vi "ScanningWaveform_v4.vi"(0 "Vy-min":dbl, 1 "Vy-max":dbl, 2 "yPixels/tPixels":dbl, 3 "xPixels/rPixels":dbl, 4 "Vx-min":dbl, 5 "Vx-max":dbl, 6 "Drawing Mode":u16(ring) items=["Image", "Fill Rectangle", "Fill Circle", "Draw Freeform", "Fill Freeform", "Ellipse Boundary", "Line"], 7 "Angle":dbl, 8 "Scanning Mode":u16(ring) items=["Raster", "Spiral"], 9 "AOrate":dbl, 10 "Points":cluster{"X":dbl, "Y":dbl}[](array[cluster]), 11 "points in ellipse":dbl) -> (12 "numPixels":dbl, 13 "Y-WaveArray":dbl[](array[numeric]), 14 "P":dbl, 19 "X-WaveArray":dbl[](array[numeric]))   [LabVIEW 2015]
uses:
  <vilib>/measure/NI_MABase.lvlib
panel:
  out "error IO":errorcluster
  out "Y Graph 4":dbl[][](graph)
  out "Y Graph 3":dbl[][](graph)
  out "X-Y Graph 3":T1(graph)
  out "Y Graph 2":dbl[](graph)
  out "X-Y Graph 2":cluster{dbl[], dbl[]}(graph)
  out "min":dbl
  out "max":dbl
  out "Points 2":cluster{"R":dbl, "Theta":dbl}[](array[cluster])
  out "X-Y Graph":cluster{dbl[], dbl[]}(graph)
  out "flyback time (us)":dbl
  out "Y Graph":dbl[](graph)
  out "X Graph":dbl[](graph)
  out "C":dbl
  out "Sx":dbl
  out "S":dbl
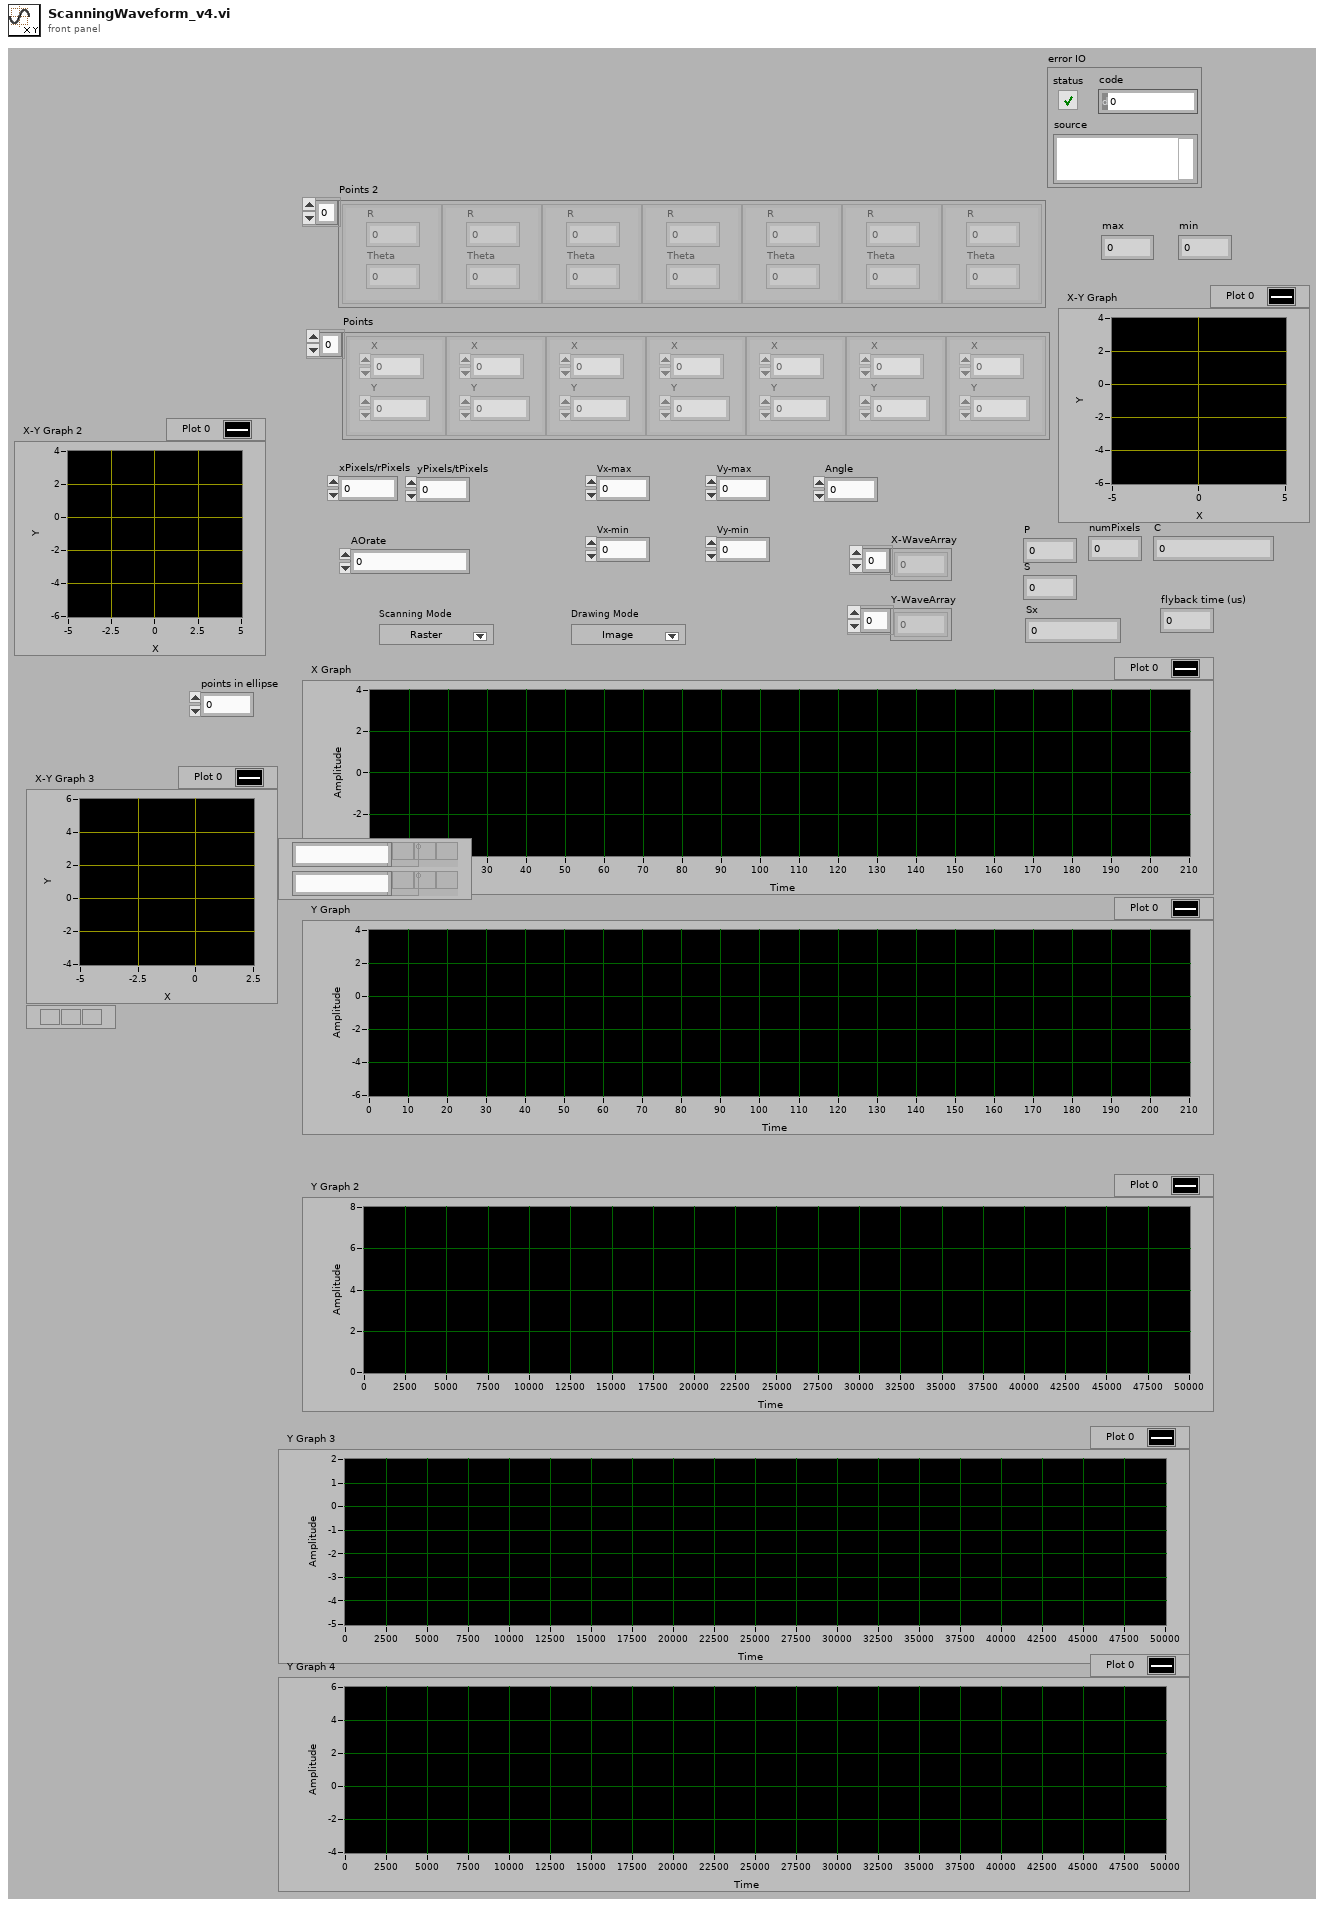
[diagram p1: front panel]
types:
  T1 = cluster{"X-WaveArray":dbl[], "Y-WaveArray":dbl[]}[]
  T2 = typedef "LVRectTypeDef.ctl" = cluster{"Left":i16, "Top":i16, "Right":i16, "Bottom":i16}
  T3 = cluster{"Xpixels":i32, "Vxminref":dbl, "Vxmaxref":dbl, "P":dbl, "Ypixels":i32, "Vyminref":dbl, "Vymaxref":dbl, "srate":sgl, "sAOxy":i32, "timeout":dbl, "type":string, "date":string, "time":string, "Colormap":u16, "Drawing Mode":u16, "Scanning Mode":u16, "square pixels":bool, "square matrix":bool, "Xpixels Img":i32, "Vx-min Img":dbl, "VX-max Img":dbl, "Ypixels Img":i32, "Vy-min Img":dbl, "Vy-max Img ":dbl, "Angle Img":dbl, "autoshutter":bool, "finite":bool, "cont":bool, "wavdet":bool, "measpoints":i32, "avpp":i32, "bufferAO":i32, "bufferAI":i32, "starttick":u32, "waveform":path, "Vx-ref":dbl, "Vy-ref":dbl, "refreshrate":dbl, "refreshbuffer":i32, "tt_cycles":i32, "motorref":refnum<k7>, "mirrorswitch":refnum<k7>, "sample mode":i32, "maxbufferAI":i32, "srateAODO":sgl, "bin":sgl, "Pel":sgl, "Angle draw":dbl, "srate Img":sgl, "ROIimg_plotbounds":T2, "auto OD":bool, "ODfilt":u16, "aAI":i32[], "aCI":i32[], "aAO":u32[], "aDO":u32[], "refwfsize":dbl, "Lifetime":bool, "Vz-Img":dbl, "Vz-ref":dbl, "Vz-reset":dbl, "AIoverride":bool, "aAS":u32[], "XYZstart":dbl[]}
  T4 = cluster{cluster{dbl, dbl}[], cluster{dbl, dbl}[]}
  T5 = cluster{"X-WaveArray":dbl[], "Y-WaveArray":dbl[]}
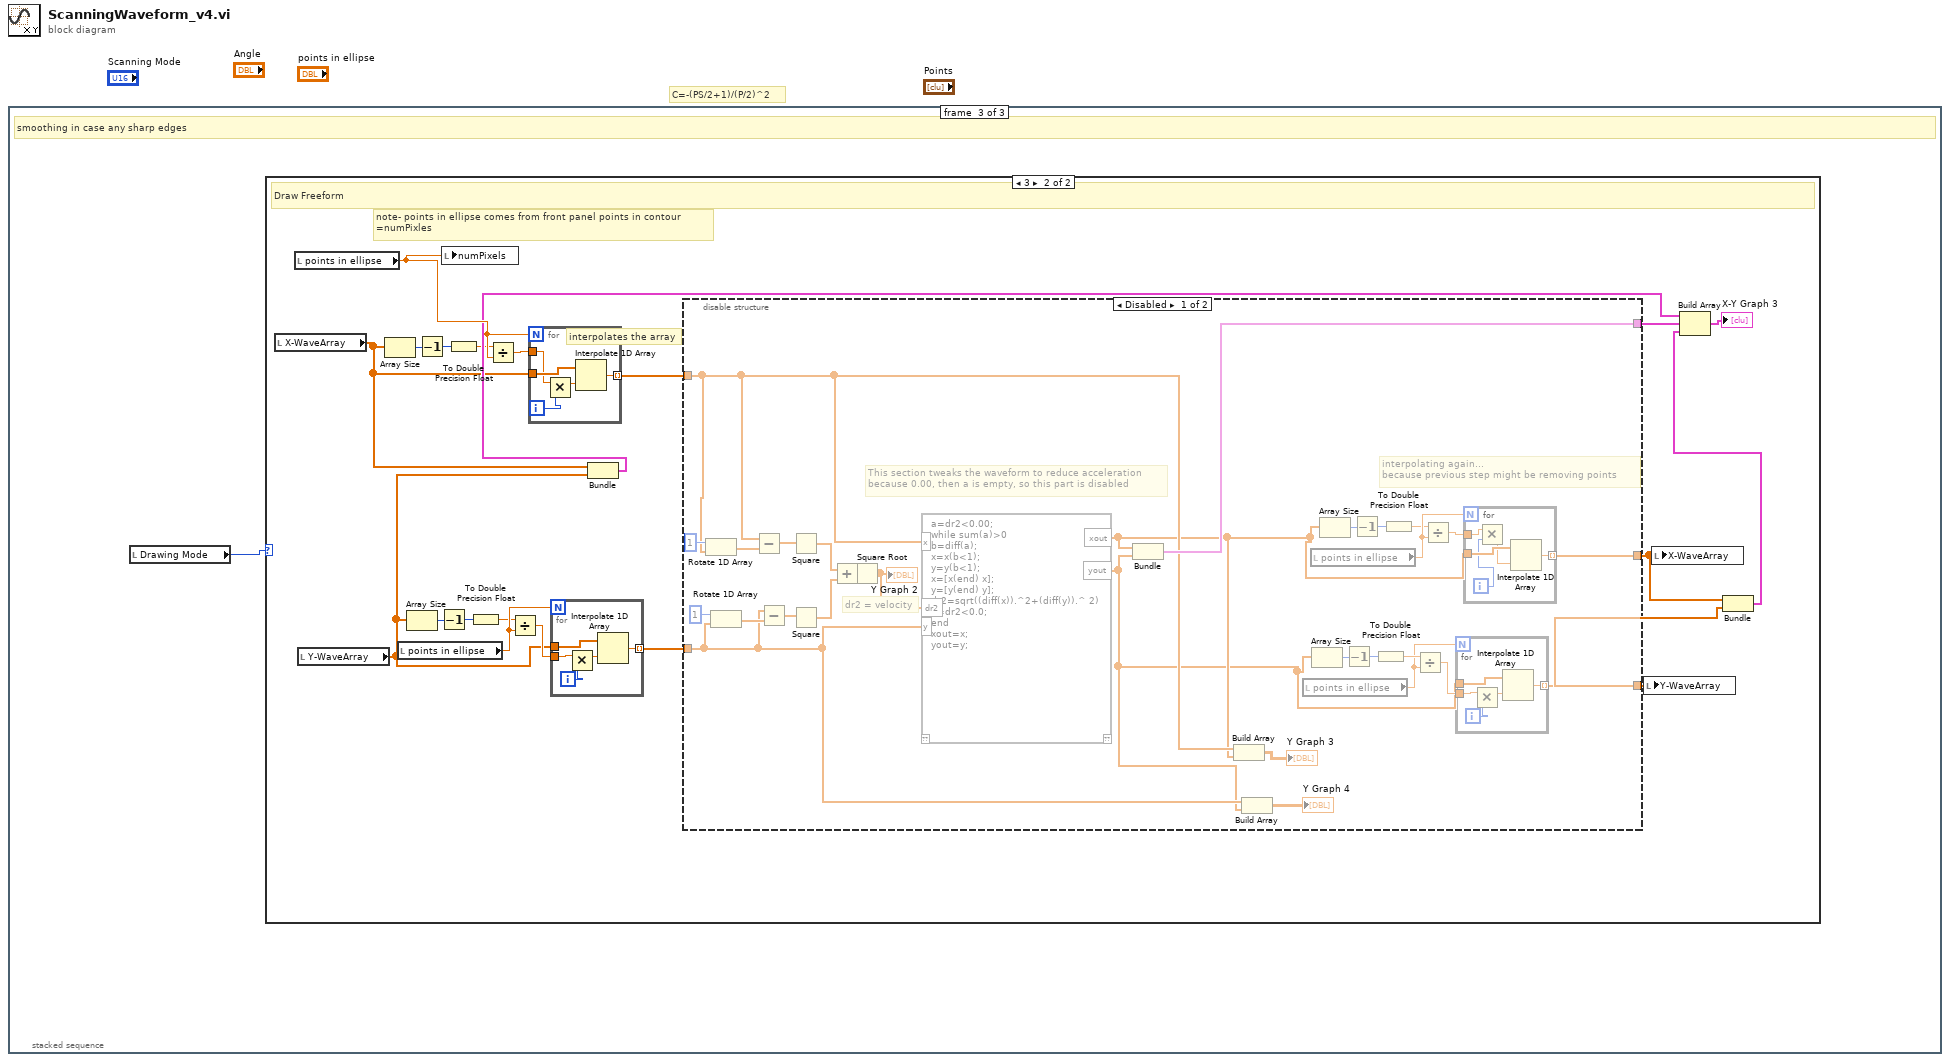
[diagram p0: block diagram]
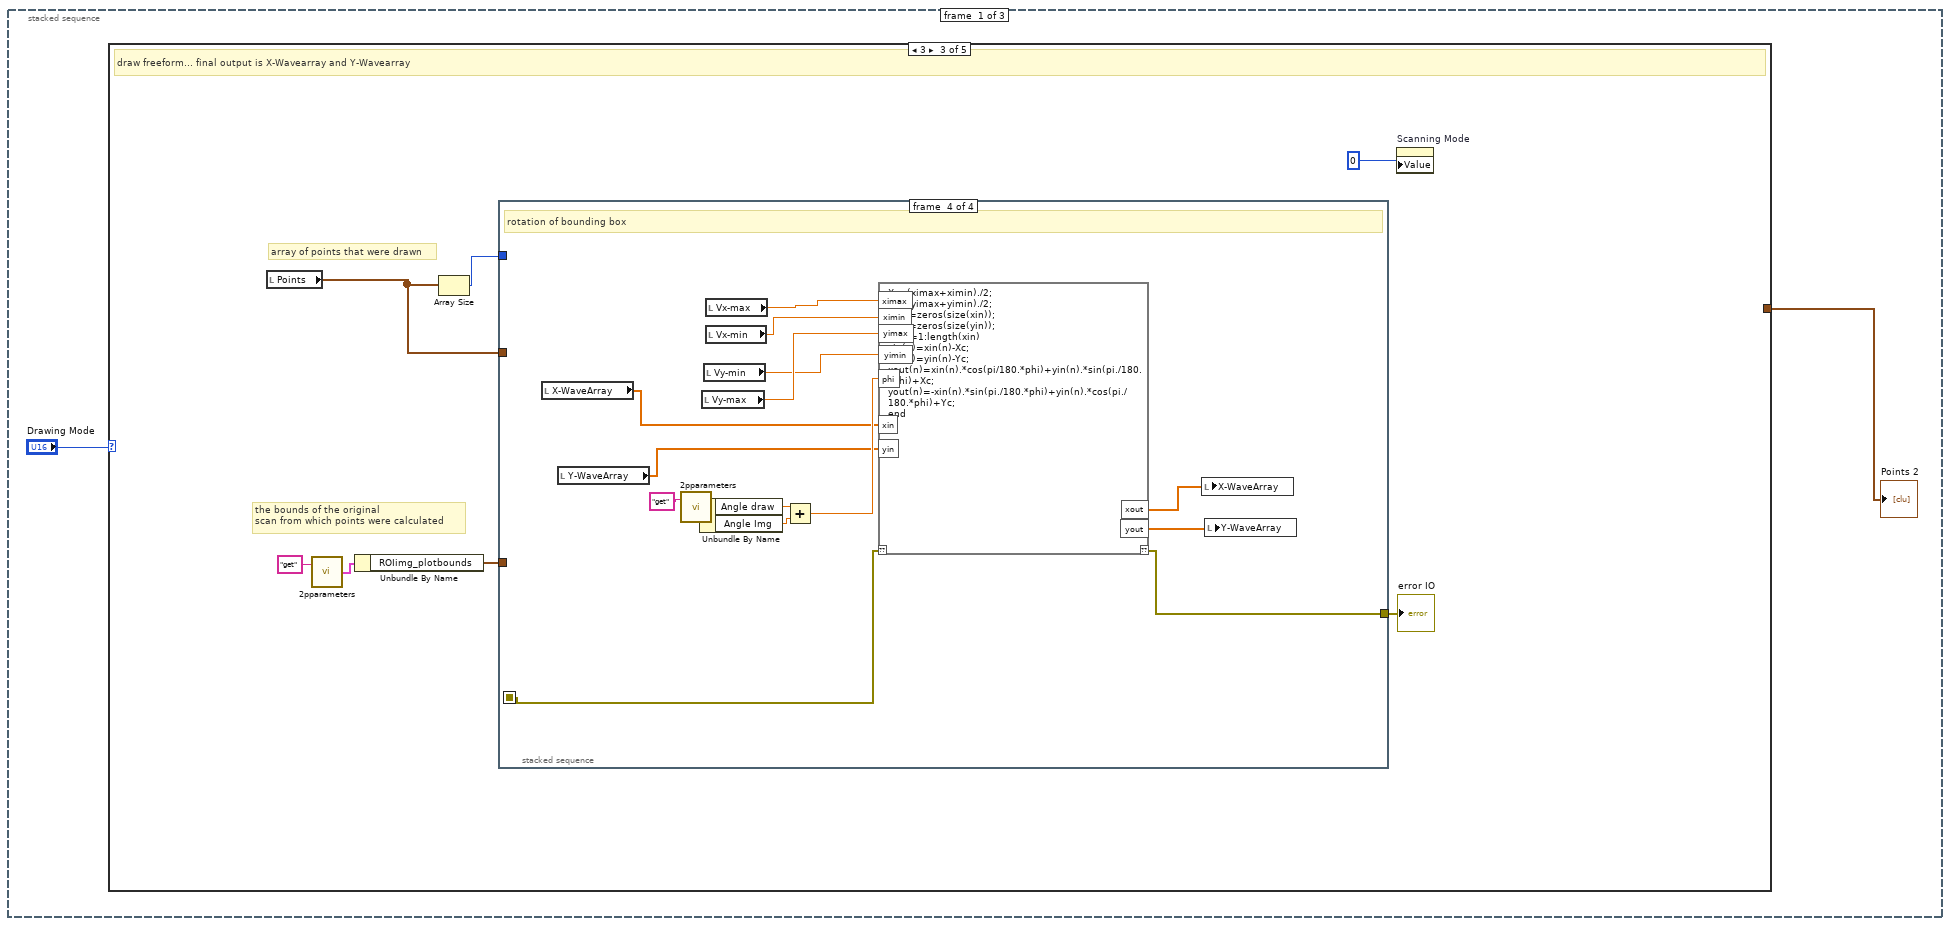
[diagram p2: hidden frame]
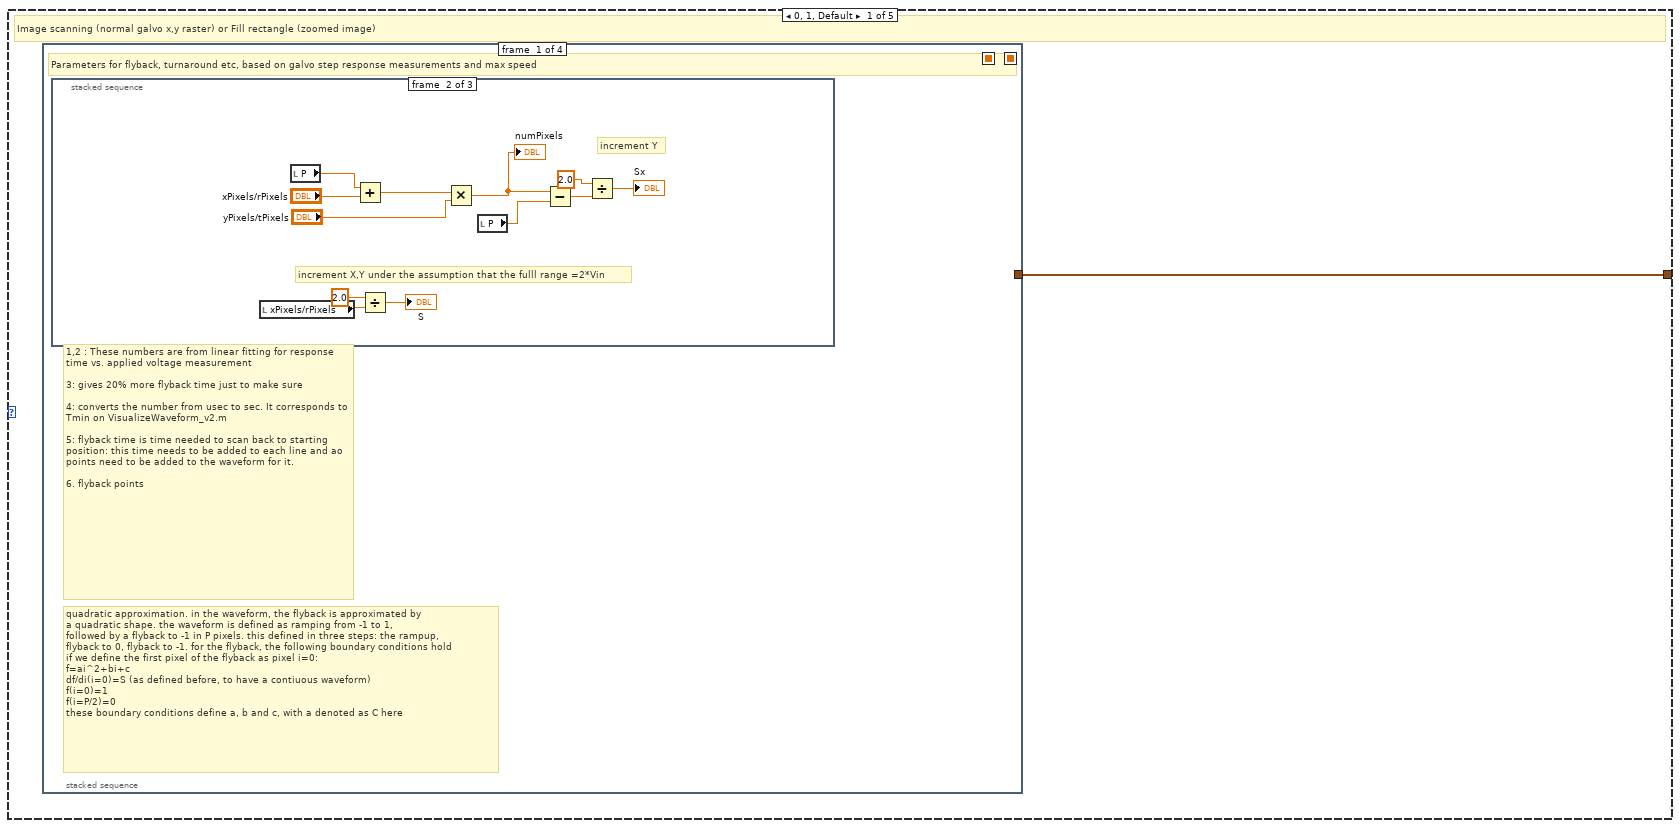
[diagram p3: hidden frame]
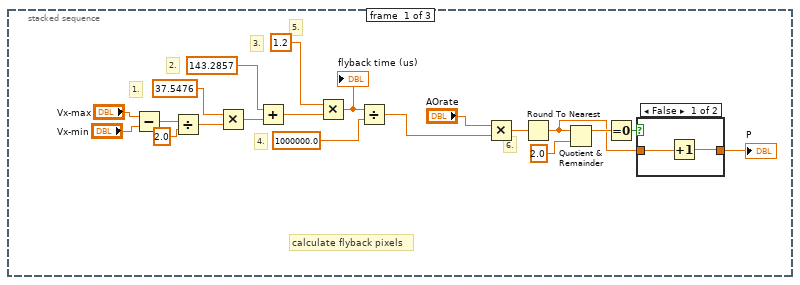
[diagram p4: hidden frame]
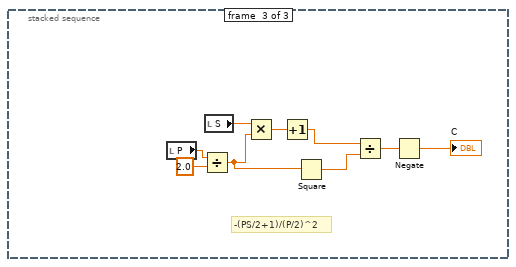
[diagram p6: hidden frame]
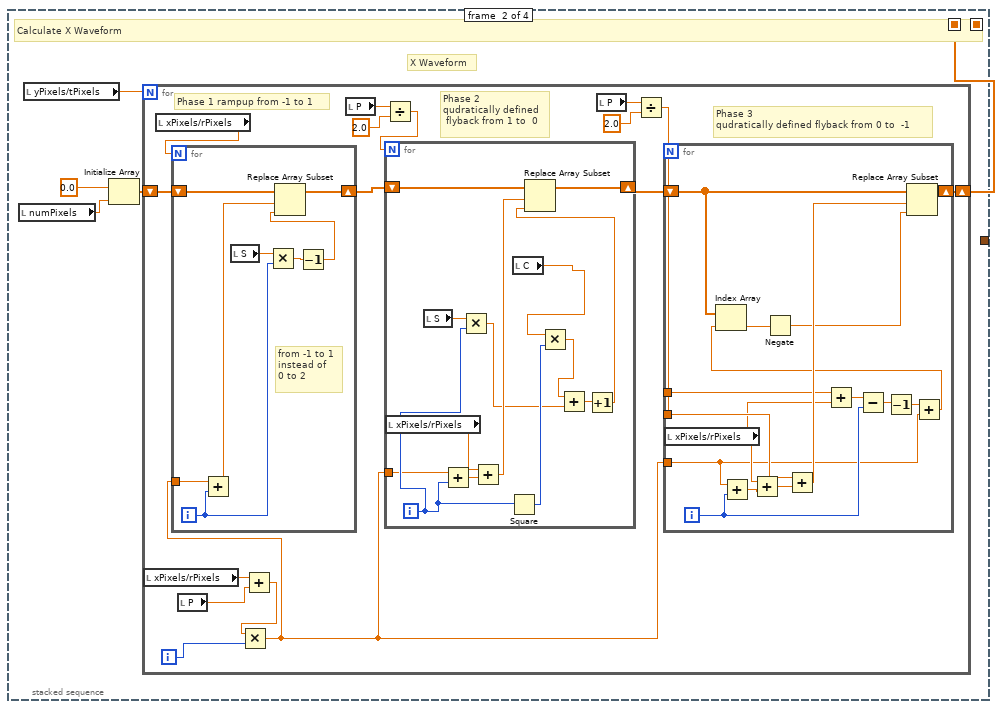
[diagram p7: hidden frame]
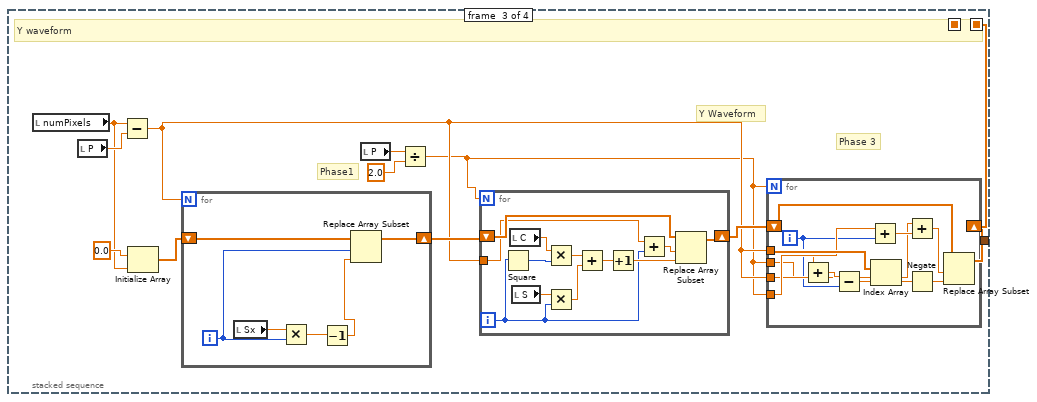
[diagram p8: hidden frame]
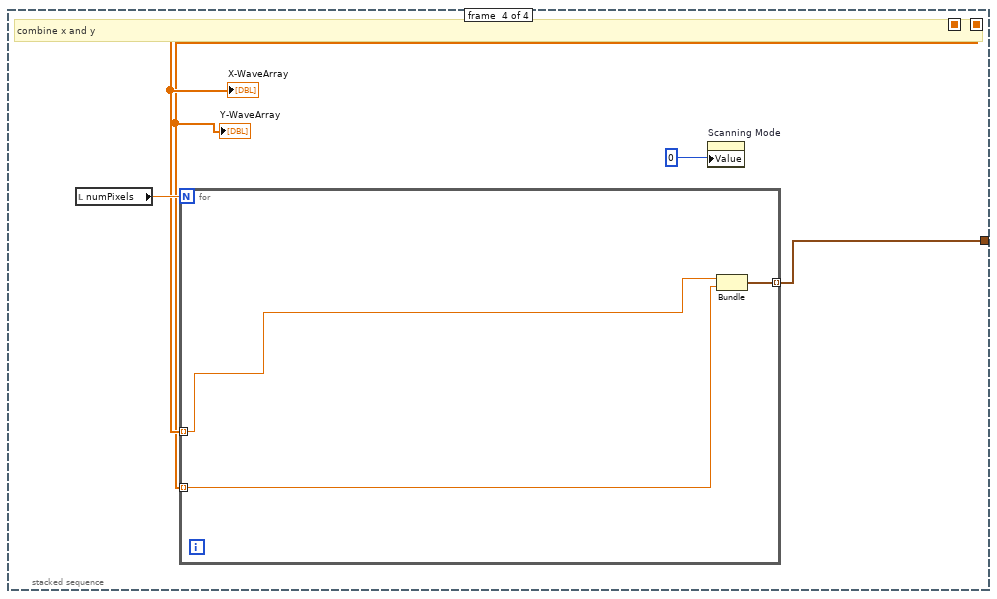
[diagram p9: hidden frame]
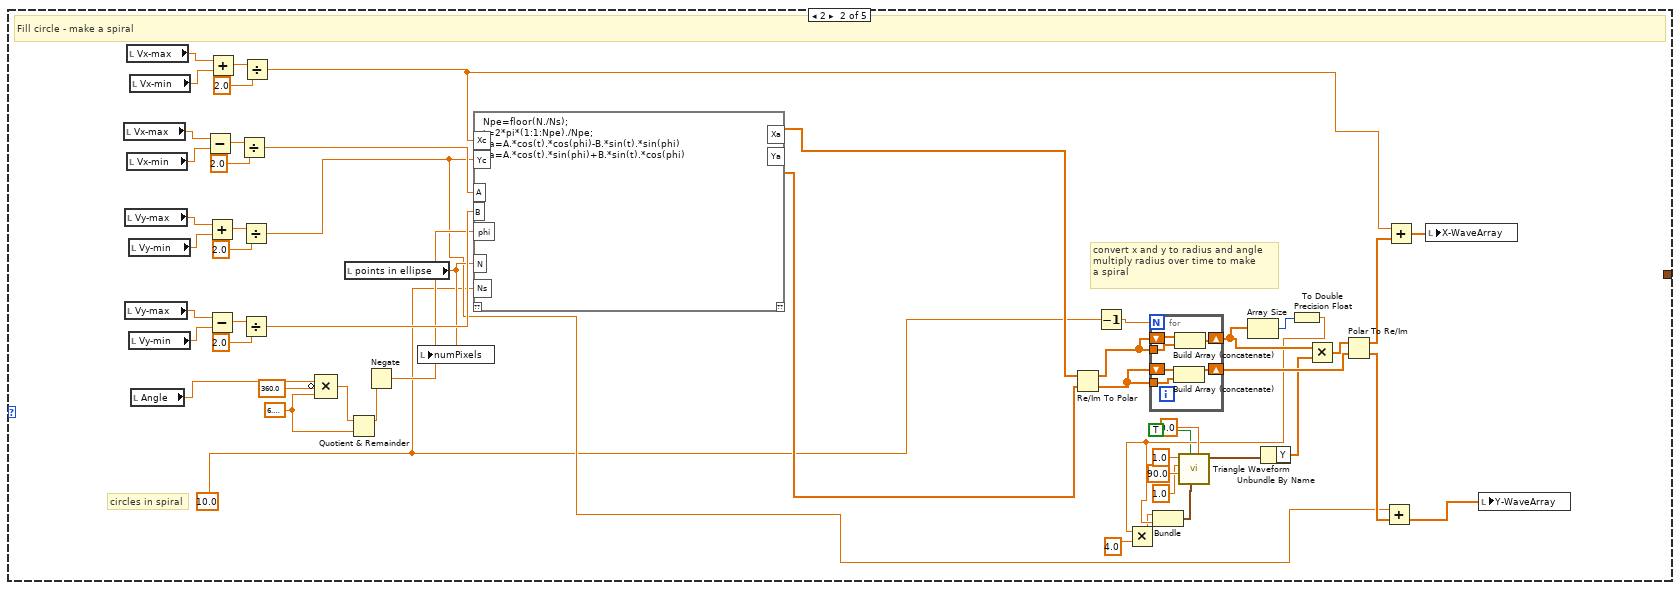
[diagram p10: hidden frame]
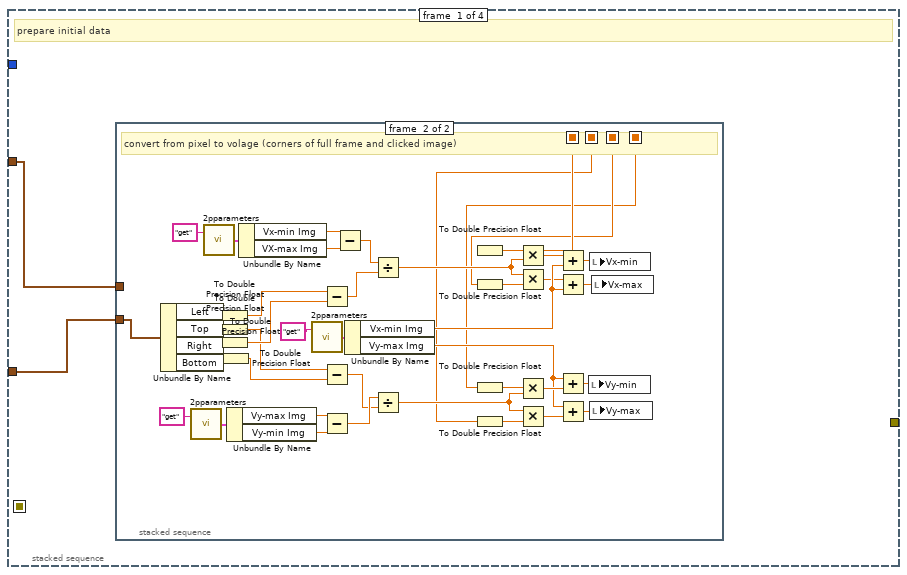
[diagram p11: hidden frame]
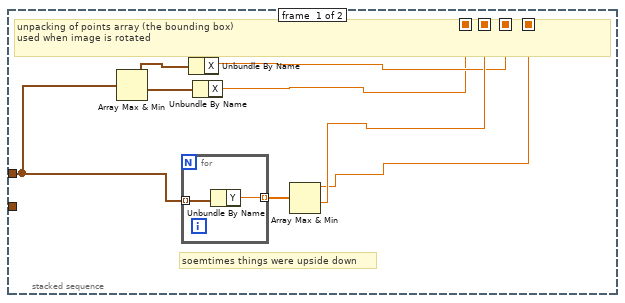
[diagram p12: hidden frame]
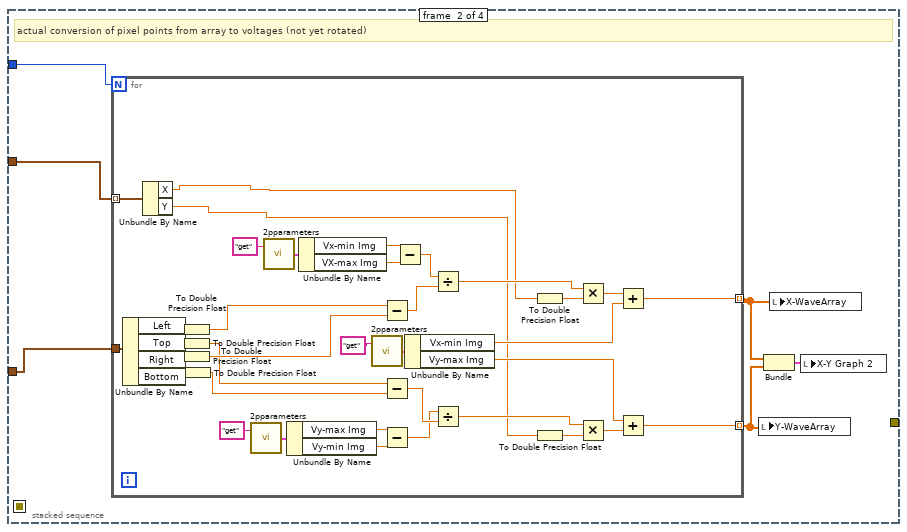
[diagram p13: hidden frame]
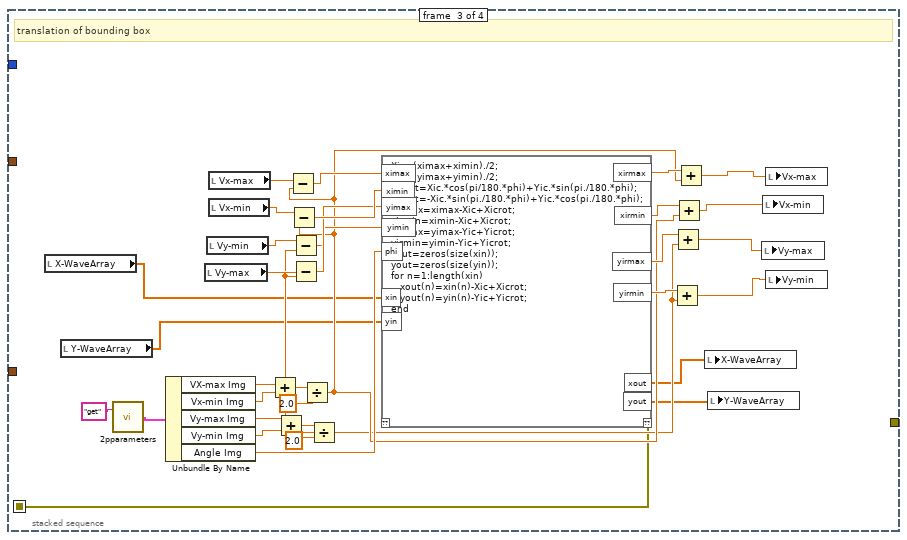
[diagram p14: hidden frame]
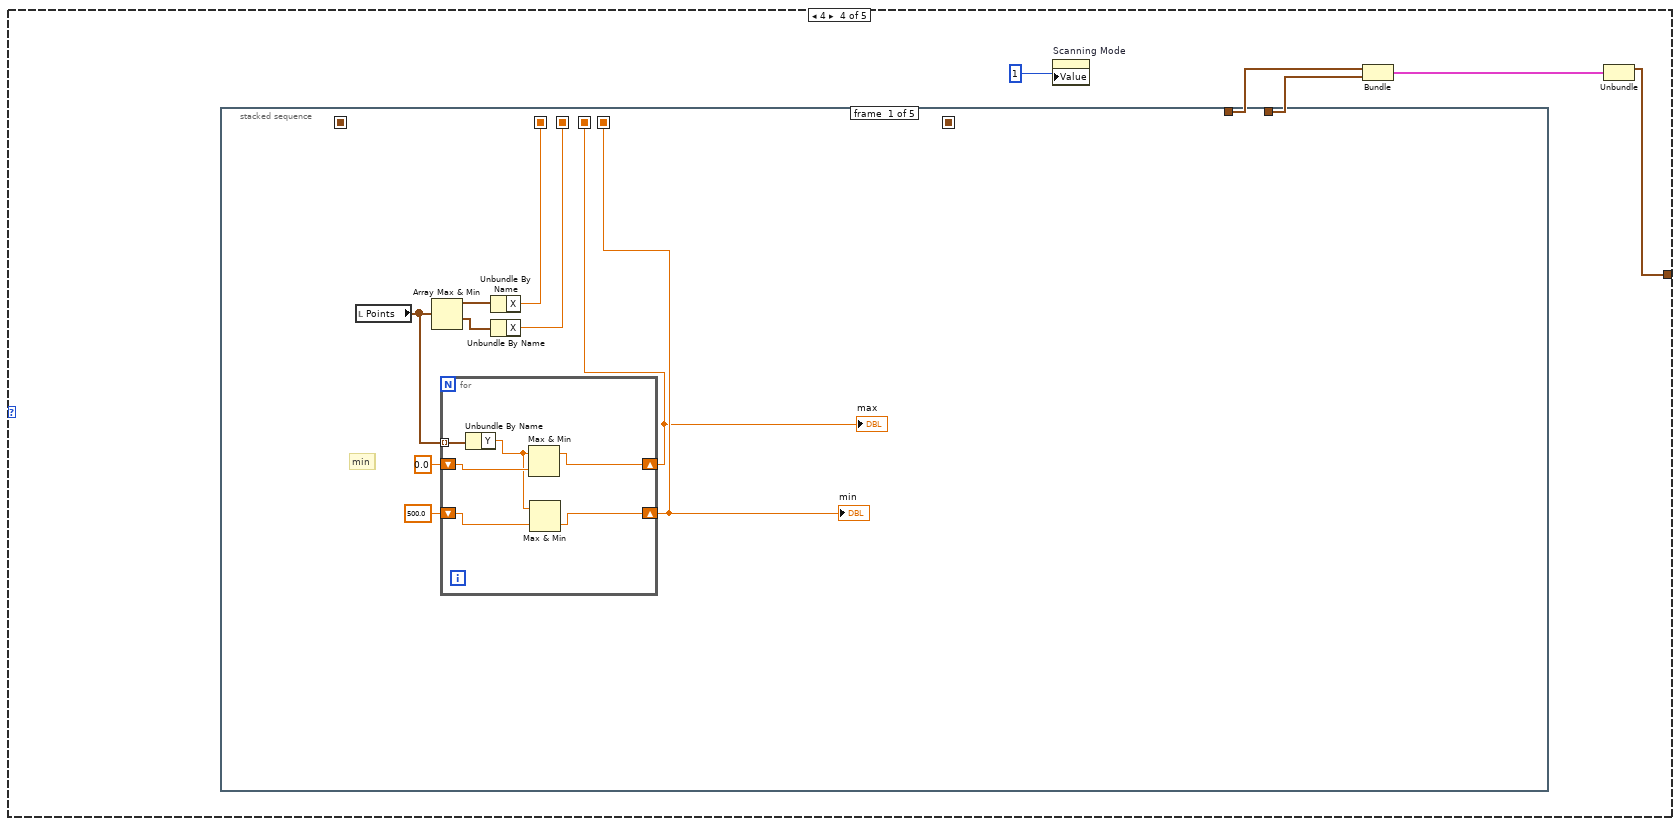
[diagram p15: hidden frame]
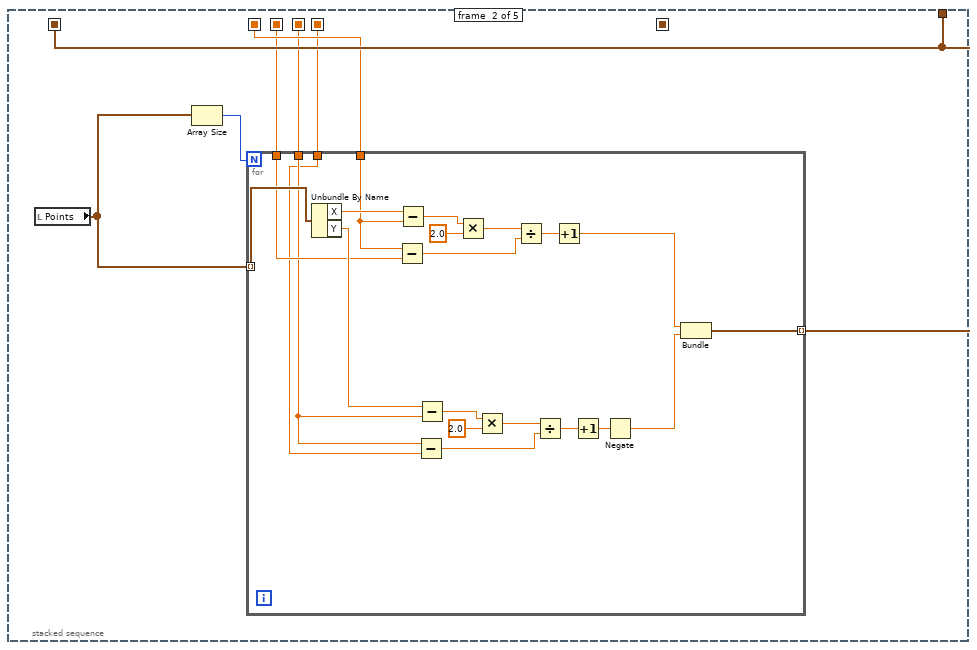
[diagram p16: hidden frame]
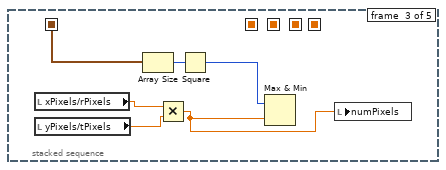
[diagram p17: hidden frame]
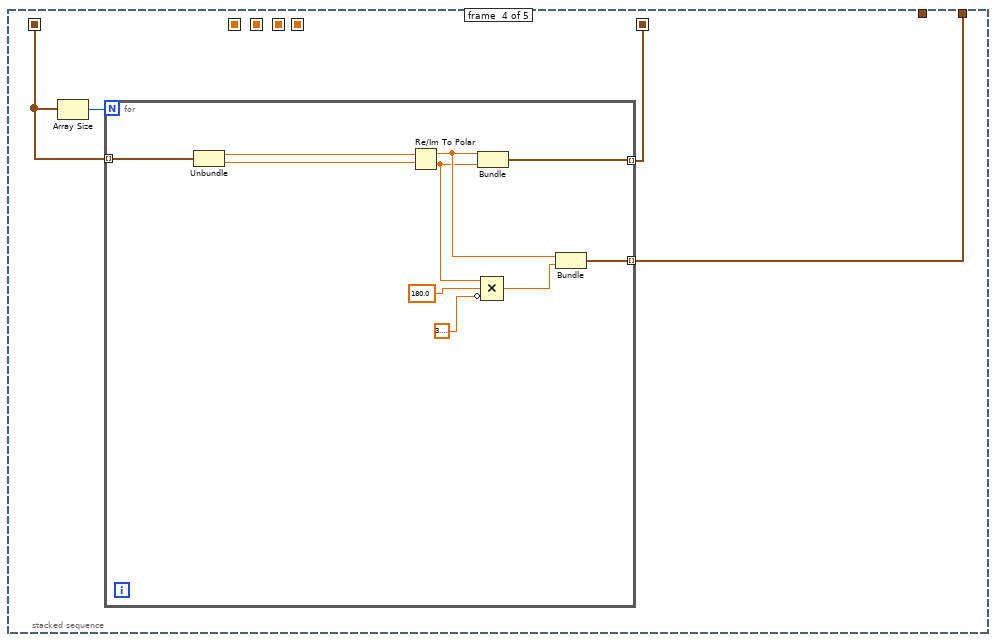
[diagram p18: hidden frame]
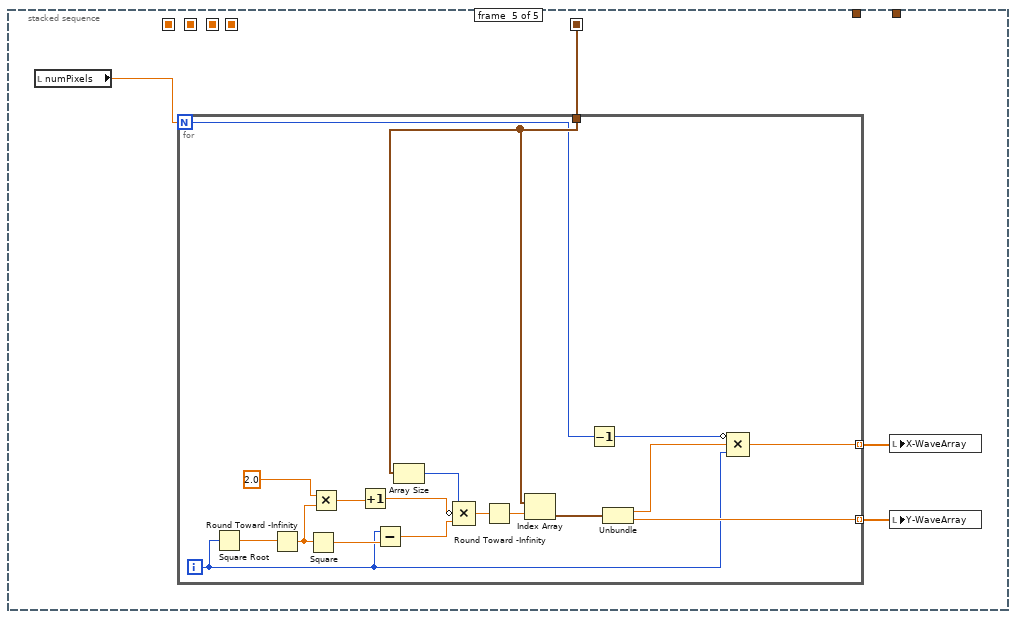
[diagram p19: hidden frame]
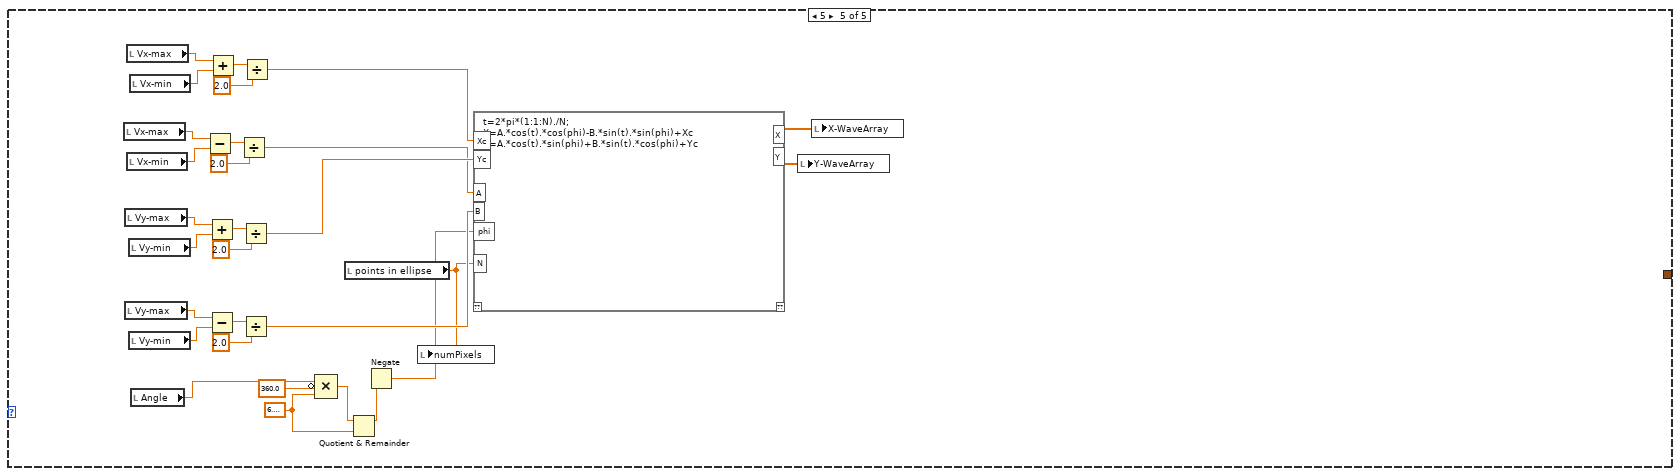
[diagram p20: hidden frame]
diagram:
  # "C=-(PS/2+1)/(P/2)^2"
  n1 = stacked-sequence {
    frame #0 {
      n2 = case shown="3" "Drawing Mode" {
        tunnel: [w3 _ _ w369 _] -> w1
        frame 0, 1, Default {
          # "Image scanning (normal galvo x,y raster) or Fill rectangle (zoomed image)"
          n3 = stacked-sequence {
            seq-local: [_ w48 _ _] -> [_ _ _ w150]
            seq-local: [_ _ w107 _] -> [_ _ _ w149]
            tunnel: [_ _ _ w151] -> w3
            frame #0 {
              # "quadratic approximation. in the waveform, the flyback is approximated by\na quadratic shape. the waveform is defined as ramping from -1 to 1, \nfollowed by a flyback to -1 in P pixels. this defined in three steps: the rampup,\nflyback to 0, flyback to -1. for the flyback, the following boundary conditions hold\nif we define the first pixel of the flyback as pixel i=0:\nf=ai^2+bi+c\ndf/di(i=0)=S (as defined before, to have a contiuous waveform)\nf(i=0)=1\nf(i=P/2)=0\nthese boundary conditions define a, b and c, with a denoted as C here"
              # "1,2 : These numbers are from linear fitting for response time vs. applied voltage measurement\n\n3: gives 20% more flyback time just to make sure\n\n4: converts the number from usec to sec. It corresponds to Tmin on VisualizeWaveform_v2.m\n\n5: flyback time is time needed to scan back to starting position: this time needs to be added to each line and ao points need to be added to the waveform for it.\n\n6. flyback points"
              # "Parameters for flyback, turnaround etc, based on galvo step response measurements and max speed"
              n4 = stacked-sequence {
                frame #0 {
                  # "calculate flyback pixels"
                  # "6."
                  # "5."
                  # "4."
                  # "3."
                  # "2."
                  # "1."
                  n5 = Subtract(x="Vx-max", y="Vx-min") -> (x-y=w5:dbl)
                  n6 = Divide(x=w5, y=2.0 ("x-y")) -> (x/y=w4:dbl)
                  n7 = Multiply(x=37.5476, y=w4) -> (x*y=w21:dbl)
                  n8 = Add(x=143.2857, y=w21) -> (x+y=w19:dbl)
                  n9 = Multiply(x=1.2, y=w19) -> (x*y=w17:dbl)
                  "flyback time (us)" <- w17
                  n10 = Divide(x=w17, y=1000000.0 ("x")) -> (x/y=w15:dbl)
                  n11 = Multiply(x="AOrate", y=w15) -> (x*y=w14:dbl)
                  n12 = Round To Nearest(number=w14) -> (nearest integer value=w9:dbl)
                  n13 = Quotient & Remainder(x=w9, y=2.0) -> (x-y*floor(x/y)=w11:dbl)  [unwired: 1 out]
                  n14 = Equal To 0?(x=w11) -> (x = 0?=w12:bool)
                  n15 = case shown="False" w12 {
                    tunnel: [w24 w26] -> w10
                    tunnel: w9 -> [w25 w26]
                    frame False {
                      n16 = Increment(x=w25) -> (x+1=w24:dbl)
                    }
                    frame True {
                    }
                  }
                  "P" <- w10
                }
                frame #1 {
                  # "increment X,Y under the assumption that the fulll range =2*Vin"
                  # "increment Y"
                  n17 = local read "xPixels/rPixels"() -> (w31:dbl)
                  n18 = local read "P"() -> (w37:dbl)
                  n19 = Add(x=w37, y="xPixels/rPixels") -> (x+y=w33:dbl)
                  n20 = Divide(x=2.0, y=w31) -> (x/y=→"S":dbl)
                  n21 = Multiply(x=w33, y="yPixels/tPixels") -> (x*y=w36:dbl)
                  "numPixels" <- w36
                  n22 = local read "P"() -> (w38:dbl)
                  n23 = Subtract(x=w36, y=w38) -> (x-y=w29:dbl)
                  n24 = Divide(x=2.0, y=w29) -> (x/y=→"Sx":dbl)
                }
                frame #2 {
                  # "-(PS/2+1)/(P/2)^2"
                  n25 = local read "P"() -> (w45:dbl)
                  n26 = Divide(x=w45, y=2.0) -> (x/y=w47:dbl)
                  n27 = local read "S"() -> (w46:dbl)
                  n28 = Multiply(x=w46, y=w47) -> (x*y=w42:dbl)
                  n29 = Increment(x=w42) -> (x+1=w39:dbl)
                  n30 = Square(x=w47) -> (x^2=w43:dbl)
                  n31 = Divide(x=w39, y=w43) -> (x/y=w44:dbl)
                  n32 = Negate(x=w44) -> (-x=→"C":dbl)
                }
              }
            }
            frame #1 {
              # "X Waveform"
              # "Calculate X Waveform"
              n33 = local read "numPixels"() -> (w50:dbl)
              n34 = local read "yPixels/tPixels"() -> (w52:dbl)
              n35 = Initialize Array(0.0 ("element"), w50) -> (w49:dbl[])
              n36 = for {
                N: w52 -> [_]
                shift-right: [w54] -> w48
                shift-left: w49 -> [w63]
                i -> [w68]
                # "Phase 3\nqudratically defined flyback from 0 to  -1"
                # "Phase 2\nqudratically defined\n flyback from 1 to  0"
                # "Phase 1 rampup from -1 to 1"
                n37 = local read "xPixels/rPixels"() -> (w67:dbl)
                n38 = local read "xPixels/rPixels"() -> (w64:dbl)
                n39 = local read "P"() -> (w66:dbl)
                n40 = Add(x=w67, y=w66) -> (x+y=w65:dbl)
                n41 = Multiply(x=w65, y=w68) -> (x*y=w53:dbl)
                n42 = for {
                  N: w64 -> [_]
                  shift-right: [w102] -> w55
                  shift-left: w63 -> [w106]
                  tunnel: w53 -> [w101]
                  i -> [w103]
                  # "from -1 to 1\ninstead of\n0 to 2"
                  n43 = Add(x=w101, y=w103) -> (x+y=w105:dbl)
                  n44 = local read "S"() -> (w104:dbl)
                  n45 = Multiply(x=w104, y=w103) -> (x*y=w100:dbl)
                  n46 = Decrement(x=w100) -> (x-1=w99:dbl)
                  n47 = Replace Array Subset(array=w106, new element=w99, index=w105) -> (w102:dbl[])
                }
                n48 = local read "P"() -> (w61:dbl)
                n49 = Divide(x=w61, y=2.0) -> (x/y=w62:dbl)
                n50 = for {
                  N: w62 -> [_]
                  shift-right: [w87] -> w57
                  shift-left: w55 -> [w98]
                  tunnel: w53 -> [w86]
                  i -> [w91]
                  n51 = local read "xPixels/rPixels"() -> (w96:dbl)
                  n52 = local read "S"() -> (w92:dbl)
                  n53 = Add(x=w86, y=w91) -> (x+y=w97:dbl)
                  n54 = Multiply(x=w92, y=w91) -> (x*y=w90:dbl)
                  n55 = Add(x=w96, y=w97) -> (x+y=w95:dbl)
                  n56 = Square(x=w91) -> (x^2=w94:i32)
                  n57 = local read "C"() -> (w85:dbl)
                  n58 = Multiply(x=w85, y=w94) -> (x*y=w93:dbl)
                  n59 = Add(x=w93, y=w90) -> (x+y=w89:dbl)
                  n60 = Increment(x=w89) -> (x+1=w88:dbl)
                  n61 = Replace Array Subset(array=w98, new element=w88, index=w95) -> (w87:dbl[])
                }
                n62 = local read "P"() -> (w58:dbl)
                n63 = Divide(x=w58, y=2.0) -> (x/y=w56:dbl)
                n64 = for {
                  N: w56 -> [_]
                  tunnel: w56 -> [w82]
                  tunnel: w56 -> [w79]
                  shift-right: [w70] -> w54
                  shift-left: w57 -> [w80]
                  tunnel: w53 -> [w69]
                  i -> [w76]
                  n65 = local read "xPixels/rPixels"() -> (w78:dbl)
                  n66 = Add(x=w69, y=w76) -> (x+y=w84:dbl)
                  n67 = Add(x=w78, y=w84) -> (x+y=w83:dbl)
                  n68 = Add(x=w82, y=w83) -> (x+y=w81:dbl)
                  n69 = Add(x=w79, y=w78) -> (x+y=w77:dbl)
                  n70 = Subtract(x=w77, y=w76) -> (x-y=w75:dbl)
                  n71 = Decrement(x=w75) -> (x-1=w74:dbl)
                  n72 = Add(x=w74, y=w69) -> (x+y=w73:dbl)
                  n73 = Index Array(array=w80, index=w73) -> (element=w72:dbl)
                  n74 = Negate(x=w72) -> (-x=w71:dbl)
                  n75 = Replace Array Subset(array=w80, new element=w71, index=w81) -> (w70:dbl[])
                }
              }
            }
            frame #2 {
              # "Phase 3"
              # "Phase1"
              # "Y Waveform"
              # "Y waveform"
              n76 = local read "numPixels"() -> (w114:dbl)
              n77 = local read "P"() -> (w115:dbl)
              n78 = Subtract(x=w114, y=w115) -> (x-y=w109:dbl)
              n79 = Initialize Array(0.0 ("element"), w114) -> (w116:dbl[])
              n80 = for {
                N: w109 -> [_]
                shift-right: [w145] -> w111
                shift-left: w116 -> [w148]
                i -> [w146]
                n81 = local read "Sx"() -> (w147:dbl)
                n82 = Multiply(x=w147, y=w146) -> (x*y=w143:dbl)
                n83 = Decrement(x=w143) -> (x-1=w144:dbl)
                n84 = Replace Array Subset(array=w148, new element=w144, index=w146) -> (w145:dbl[])
              }
              n85 = local read "P"() -> (w113:dbl)
              n86 = Divide(x=w113, y=2.0) -> (x/y=w108:dbl)
              n87 = for {
                N: w108 -> [_]
                shift-right: [w135] -> w110
                shift-left: w111 -> [w142]
                tunnel: w109 -> [w134]
                i -> [w132]
                n88 = Square(x=w132) -> (x^2=w140:i32)
                n89 = local read "C"() -> (w131:dbl)
                n90 = local read "S"() -> (w133:dbl)
                n91 = Multiply(x=w131, y=w140) -> (x*y=w139:dbl)
                n92 = Multiply(x=w133, y=w132) -> (x*y=w138:dbl)
                n93 = Add(x=w139, y=w138) -> (x+y=w137:dbl)
                n94 = Increment(x=w137) -> (x+1=w136:dbl)
                n95 = Add(x=w134, y=w132) -> (x+y=w141:dbl)
                n96 = Replace Array Subset(array=w142, new element=w136, index=w141) -> (w135:dbl[])
              }
              n97 = for {
                N: w108 -> [_]
                shift-right: [w124] -> w107
                shift-left: w110 -> [w128]
                tunnel: w108 -> [w123]
                tunnel: w109 -> [w122]
                tunnel: w109 -> [w121]
                tunnel: w108 -> [w120]
                i -> [w118]
                n98 = Add(x=w121, y=w120) -> (x+y=w127:dbl)
                n99 = Subtract(x=w127, y=w118) -> (x-y=w119:dbl)
                n100 = Add(x=w123, y=w118) -> (x+y=w130:dbl)
                n101 = Index Array(array=w128, index=w119) -> (element=w126:dbl)
                n102 = Add(x=w122, y=w130) -> (x+y=w129:dbl)
                n103 = Negate(x=w126) -> (-x=w125:dbl)
                n104 = Replace Array Subset(array=w128, new element=w125, index=w129) -> (w124:dbl[])
              }
            }
            frame #3 {
              # "combine x and y"
              n105 = local read "numPixels"() -> (w153:dbl)
              n106 = for {
                N: w153 -> [_]
                tunnel: w150 -> [w155] mode=indexing
                tunnel: w149 -> [w154] mode=indexing
                tunnel: [w156] -> w151 mode=indexing
                n107 = Bundle("element"=w155, "element"=w154) -> (w156:cluster{"element":dbl, "element":dbl})  [unwired: 1 in]
              }
              n108 = property on="Scanning Mode" class="Ring (strict)"("Value"=0) -> ()  [unwired: 2 in, 2 out]
              "X-WaveArray" <- w150
              "Y-WaveArray" <- w149
            }
          }
        }
        frame 2 {
          w159 = 10.0 ("cycles in spiral")
          w188 = 6.283185307179586
          # "convert x and y to radius and angle\nmultiply radius over time to make\na spiral"
          # "circles in spiral"
          # "Fill circle - make a spiral"
          n109 = local read "Vx-max"() -> (w197:dbl)
          n110 = local read "Vy-max"() -> (w201:dbl)
          n111 = local read "Vy-max"() -> (w196:dbl)
          n112 = local read "Vx-max"() -> (w208:dbl)
          n113 = local read "Vx-min"() -> (w198:dbl)
          n114 = local read "Vy-min"() -> (w202:dbl)
          n115 = local read "Vy-min"() -> (w195:dbl)
          n116 = local read "Vx-min"() -> (w207:dbl)
          n117 = local read "Angle"() -> (w186:dbl)
          n118 = Subtract(x=w197, y=w198) -> (x-y=w199:dbl)
          n119 = Add(x=w201, y=w202) -> (x+y=w203:dbl)
          n120 = Subtract(x=w196, y=w195) -> (x-y=w194:dbl)
          n121 = Add(x=w208, y=w207) -> (x+y=w206:dbl)
          n122 = Divide(x=w199, y=2.0) -> (x/y=w192:dbl)
          n123 = Divide(x=w203, y=2.0) -> (x/y=w160:dbl)
          n124 = Divide(x=w194, y=2.0) -> (x/y=w191:dbl)
          n125 = Divide(x=w206, y=2.0) -> (x/y=w162:dbl)
          n126 = Compound Arithmetic op=MULTIPLY(w186, invert 360.0, w188) -> (w189:dbl)
          n127 = local read "points in ellipse"() -> (w190:dbl)
          n128 = Quotient & Remainder(x=w189, y=w188) -> (x-y*floor(x/y)=w185:dbl)  [unwired: 1 out]
          n129 = Negate(x=w185) -> (-x=w184:dbl)
          n130 = local write "numPixels"(w190) -> ()
          n131 = script code="Npe=floor(N./Ns);\nt=2*pi*(1:1:Npe)./Npe;\nXa=A.*cos(t).*cos(phi)-B.*sin(t).*sin(phi)\nYa=A.*cos(t).*sin(phi)+B.*sin(t).*cos(phi)"("Xc"=w162, "Yc"=w160, "A"=w192, "B"=w191, "phi"=w184, "N"=w190, "Ns"=w159) -> ("Xa"=w163:dbl[], "Ya"=w161:dbl[])  [unwired: 1 in, 1 out]
          n132 = Re/Im To Polar(2:w161, 3:w163) -> (0:w181:dbl[], 1:w182:dbl[])
          n133 = Decrement(x=w159) -> (x-1=w183:dbl)
          n134 = for {
            N: w183 -> [_]
            shift-right: [w212] -> w173
            shift-left: w182 -> [w213]
            tunnel: w182 -> [w214]
            shift-right: [w209] -> w171
            shift-left: w181 -> [w211]
            tunnel: w181 -> [w210]
            n135 = Build Array (concatenate)(w211, w210) -> (w209:dbl[])
            n136 = Build Array (concatenate)(w213, w214) -> (w212:dbl[])
          }
          n137 = Array Size(array=w173) -> (size(s)=w179:i32)
          n138 = To Double Precision Float(number=w179) -> (double precision float=w166:dbl)
          n139 = Multiply(x=w166, y=4.0) -> (x*y=w165:dbl)
          n140 = Bundle(w165, w166) -> (w177:cluster{dbl, dbl})  [unwired: 1 in]
          n141 = call <vilib>:"Triangle Waveform.vi"("offset"=0.0, "sampling info"=w177, "reset signal"=TRUE, "phase"=90.0, "amplitude"=1.0, "frequency"=1.0) -> ("signal out"=w167:waveform(dbl))  [unwired: 4 in, 1 out]
          n142 = Unbundle By Name(w167) -> ("Y"=w168:dbl[])
          n143 = Multiply(x=w173, y=w168) -> (x*y=w172:dbl[])
          n144 = Polar To Re/Im(2:w171, 3:w172) -> (0:w170:dbl[], 1:w169:dbl[])
          n145 = Add(x=w160, y=w170) -> (x+y=w158:dbl[])
          n146 = Add(x=w162, y=w169) -> (x+y=w157:dbl[])
          n147 = local write "X-WaveArray"(w157) -> ()
          n148 = local write "Y-WaveArray"(w158) -> ()
        }
        frame 3 {
          # "the bounds of the original \nscan from which points were calculated"
          # "array of points that were drawn"
          # "draw freeform... final output is X-Wavearray and Y-Wavearray"
          n149 = local read "Points"() -> (w218:cluster{"X":dbl, "Y":dbl}[])
          n150 = call "2pparameters.vi"("command"="get") -> ("params out"=w216:T3)  [unwired: 1 in]
          n151 = Unbundle By Name(w216) -> ("ROIimg_plotbounds"=w217:T2)
          n152 = Array Size(array=w218) -> (size(s)=w219:i32)
          n153 = stacked-sequence {
            seq-local: [_ _ w319 _] -> [_ _ _ w354]
            tunnel: w218 -> [w222 w281 _ _]
            tunnel: w217 -> [w223 w282 _ _]
            tunnel: w219 -> [_ w280 _ _]
            tunnel: [_ _ _ w353] -> w215
            frame #0 {
              # "prepare initial data"
              n154 = stacked-sequence {
                seq-local: [w224 _] -> [_ w238]
                seq-local: [w227 _] -> [_ w237]
                seq-local: [w225 _] -> [_ w236]
                seq-local: [w226 _] -> [_ w235]
                tunnel: w222 -> [w231 _]
                tunnel: w223 -> [_ w234]
                frame #0 {
                  # "soemtimes things were upside down"
                  # "unpacking of points array (the bounding box)\nused when image is rotated"
                  n155 = Array Max & Min(array=w231) -> (max value=w230:cluster{"X":dbl, "Y":dbl}, min value=w229:cluster{"X":dbl, "Y":dbl})  [unwired: 2 out]
                  n156 = for {
                    tunnel: w231 -> [w233] mode=indexing
                    tunnel: [w232] -> w228 mode=indexing
                    n157 = Unbundle By Name(w233) -> ("Y"=w232:dbl)
                  }
                  n158 = Unbundle By Name(w230) -> ("X"=w225:dbl)
                  n159 = Unbundle By Name(w229) -> ("X"=w224:dbl)
                  n160 = Array Max & Min(array=w228) -> (max value=w226:dbl, min value=w227:dbl)  [unwired: 2 out]
                }
                frame #1 {
                  # "convert from pixel to volage (corners of full frame and clicked image)"
                  n161 = Unbundle By Name(w234) -> ("Left"=w239:i16, "Top"=w240:i16, "Right"=w241:i16, "Bottom"=w242:i16)
                  n162 = call "2pparameters.vi"("command"="get") -> ("params out"=w260:T3)  [unwired: 1 in]
                  n163 = call "2pparameters.vi"("command"="get") -> ("params out"=w248:T3)  [unwired: 1 in]
                  n164 = To Double Precision Float(number=w239) -> (double precision float=w275:dbl)
                  n165 = To Double Precision Float(number=w240) -> (double precision float=w243:dbl)
                  n166 = To Double Precision Float(number=w241) -> (double precision float=w276:dbl)
                  n167 = To Double Precision Float(number=w242) -> (double precision float=w244:dbl)
                  n168 = Unbundle By Name(w260) -> ("Vy-max Img"=w262:dbl, "Vy-min Img"=w263:dbl)
                  n169 = Unbundle By Name(w248) -> ("Vx-min Img"=w254:dbl, "VX-max Img"=w249:dbl)
                  n170 = call "2pparameters.vi"("command"="get") -> ("params out"=w253:T3)  [unwired: 1 in]
                  n171 = Subtract(x=w275, y=w276) -> (x-y=w245:dbl)
                  n172 = Subtract(x=w243, y=w244) -> (x-y=w246:dbl)
                  n173 = Subtract(x=w262, y=w263) -> (x-y=w264:dbl)
                  n174 = Subtract(x=w254, y=w249) -> (x-y=w250:dbl)
                  n175 = Unbundle By Name(w253) -> ("Vx-min Img"=w258:dbl, "Vy-max Img"=w266:dbl)
                  n176 = Divide(x=w250, y=w245) -> (x/y=w272:dbl)
                  n177 = Divide(x=w264, y=w246) -> (x/y=w273:dbl)
                  n178 = To Double Precision Float(number=w238) -> (double precision float=w271:dbl)
                  n179 = To Double Precision Float(number=w236) -> (double precision float=w256:dbl)
                  n180 = To Double Precision Float(number=w235) -> (double precision float=w265:dbl)
                  n181 = To Double Precision Float(number=w237) -> (double precision float=w274:dbl)
                  n182 = Multiply(x=w271, y=w272) -> (x*y=w255:dbl)
                  n183 = Multiply(x=w272, y=w256) -> (x*y=w257:dbl)
                  n184 = Multiply(x=w265, y=w273) -> (x*y=w267:dbl)
                  n185 = Multiply(x=w273, y=w274) -> (x*y=w268:dbl)
                  n186 = Add(x=w255, y=w258) -> (x+y=w251:dbl)
                  n187 = Add(x=w257, y=w258) -> (x+y=w259:dbl)
                  n188 = Add(x=w266, y=w267) -> (x+y=w269:dbl)
                  n189 = Add(x=w266, y=w268) -> (x+y=w270:dbl)
                  n190 = local write "Vy-min"(w269) -> ()
                  n191 = local write "Vx-min"(w251) -> ()
                  n192 = local write "Vy-max"(w270) -> ()
                  n193 = local write "Vx-max"(w259) -> ()
                }
              }
            }
            frame #1 {
              # "actual conversion of pixel points from array to voltages (not yet rotated)"
              n194 = for {
                N: w280 -> [_]
                tunnel: w282 -> [w290]
                tunnel: w281 -> [w289] mode=indexing
                tunnel: [w286] -> w278 mode=indexing
                tunnel: [w285] -> w277 mode=indexing
                n195 = Unbundle By Name(w290) -> ("Left"=w318:i16, "Top"=w317:i16, "Right"=w316:i16, "Bottom"=w315:i16)
                n196 = Unbundle By Name(w289) -> ("X"=w284:dbl, "Y"=w283:dbl)
                n197 = To Double Precision Float(number=w318) -> (double precision float=w288:dbl)
                n198 = To Double Precision Float(number=w317) -> (double precision float=w287:dbl)
                n199 = To Double Precision Float(number=w316) -> (double precision float=w291:dbl)
                n200 = To Double Precision Float(number=w315) -> (double precision float=w314:dbl)
                n201 = call "2pparameters.vi"("command"="get") -> ("params out"=w301:T3)  [unwired: 1 in]
                n202 = call "2pparameters.vi"("command"="get") -> ("params out"=w310:T3)  [unwired: 1 in]
                n203 = Unbundle By Name(w301) -> ("Vy-max Img"=w299:dbl, "Vy-min Img"=w298:dbl)
                n204 = Unbundle By Name(w310) -> ("Vx-min Img"=w305:dbl, "VX-max Img"=w309:dbl)
                n205 = call "2pparameters.vi"("command"="get") -> ("params out"=w306:T3)  [unwired: 1 in]
                n206 = Subtract(x=w288, y=w291) -> (x-y=w313:dbl)
                n207 = Subtract(x=w287, y=w314) -> (x-y=w312:dbl)
                n208 = Subtract(x=w299, y=w298) -> (x-y=w297:dbl)
                n209 = Subtract(x=w305, y=w309) -> (x-y=w308:dbl)
                n210 = Unbundle By Name(w306) -> ("Vx-min Img"=w302:dbl, "Vy-max Img"=w296:dbl)
                n211 = Divide(x=w308, y=w313) -> (x/y=w294:dbl)
                n212 = Divide(x=w297, y=w312) -> (x/y=w293:dbl)
                n213 = To Double Precision Float(number=w284) -> (double precision float=w304:dbl)
                n214 = To Double Precision Float(number=w283) -> (double precision float=w292:dbl)
                n215 = Multiply(x=w294, y=w304) -> (x*y=w303:dbl)
                n216 = Multiply(x=w293, y=w292) -> (x*y=w295:dbl)
                n217 = Add(x=w303, y=w302) -> (x+y=w286:dbl)
                n218 = Add(x=w296, y=w295) -> (x+y=w285:dbl)
              }
              n219 = local write "Y-WaveArray"(w277) -> ()
              n220 = Bundle(w278, w277) -> (w279:cluster{dbl[], dbl[]})  [unwired: 1 in]
              n221 = local write "X-WaveArray"(w278) -> ()
              n222 = local write "X-Y Graph 2"(w279) -> ()
            }
            frame #2 {
              # "translation of bounding box"
              n223 = local read "X-WaveArray"() -> (w322:dbl[])
              n224 = local read "Y-WaveArray"() -> (w323:dbl[])
              n225 = call "2pparameters.vi"("command"="get") -> ("params out"=w335:T3)  [unwired: 1 in]
              n226 = Unbundle By Name(w335) -> ("VX-max Img"=w337:dbl, "Vx-min Img"=w338:dbl, "Vy-max Img"=w339:dbl, "Vy-min Img"=w340:dbl, "Angle Img"=w330:dbl)
              n227 = local read "Vy-max"() -> (w347:dbl)
              n228 = local read "Vy-min"() -> (w348:dbl)
              n229 = local read "Vx-max"() -> (w345:dbl)
              n230 = local read "Vx-min"() -> (w346:dbl)
              n231 = Add(x=w337, y=w338) -> (x+y=w341:dbl)
              n232 = Add(x=w339, y=w340) -> (x+y=w344:dbl)
              n233 = Divide(x=w341, y=2.0) -> (x/y=w325:dbl)
              n234 = Subtract(x=w345, y=w325) -> (x-y=w334:dbl)
              n235 = Subtract(x=w346, y=w325) -> (x-y=w333:dbl)
              n236 = Divide(x=w344, y=2.0) -> (x/y=w324:dbl)
              n237 = Subtract(x=w348, y=w324) -> (x-y=w331:dbl)
              n238 = Subtract(x=w347, y=w324) -> (x-y=w332:dbl)
              n239 = script code="Xic=(ximax+ximin)./2;\nYic=(yimax+yimin)./2;\nXicrot=Xic.*cos(pi/180.*phi)+Yic.*sin(pi./180.*phi);\nYicrot=-Xic.*sin(pi./180.*phi)+Yic.*cos(pi./180.*phi);\nxirmax=ximax-Xic+Xicrot;\nxirmin=ximin-Xic+Xicrot;\nyirmax=yimax-Yic+Yicrot;\nyirmin=yimin-Yic+Yicrot;\nxout=zeros(size(xin));\nyout=zeros(size(yin));\nfor n=1:length(xin)\n   xout(n)=xin(n)-Xic+Xicrot;\n   yout(n)=yin(n)-Yic+Yicrot;\nend"("ximax"=w334, "ximin"=w333, "yimax"=w332, "yimin"=w331, "phi"=w330, "xin"=w322, "yin"=w323) -> ("??"=w319:errorcluster, "xirmax"=w329:dbl, "xirmin"=w328:dbl, "yirmax"=w327:dbl, "yirmin"=w326:dbl, "xout"=w321:dbl[], "yout"=w320:dbl[])  [unwired: 1 in]
              n240 = Add(x=w326, y=w324) -> (x+y=w352:dbl)
              n241 = Add(x=w327, y=w324) -> (x+y=w351:dbl)
              n242 = Add(x=w328, y=w325) -> (x+y=w350:dbl)
              n243 = Add(x=w329, y=w325) -> (x+y=w349:dbl)
              n244 = local write "X-WaveArray"(w321) -> ()
              n245 = local write "Y-WaveArray"(w320) -> ()
              n246 = local write "Vy-max"(w351) -> ()
              n247 = local write "Vx-min"(w350) -> ()
              n248 = local write "Vx-max"(w349) -> ()
              n249 = local write "Vy-min"(w352) -> ()
            }
            frame #3 {
              # "rotation of bounding box"
              n250 = local read "X-WaveArray"() -> (w357:dbl[])
              n251 = local read "Y-WaveArray"() -> (w358:dbl[])
              n252 = call "2pparameters.vi"("command"="get") -> ("params out"=w364:T3)  [unwired: 1 in]
              n253 = Unbundle By Name(w364) -> ("Angle draw"=w365:dbl, "Angle Img"=w366:dbl)
              n254 = local read "Vy-max"() -> (w362:dbl)
              n255 = local read "Vy-min"() -> (w361:dbl)
              n256 = local read "Vx-max"() -> (w359:dbl)
              n257 = local read "Vx-min"() -> (w360:dbl)
              n258 = Add(x=w365, y=w366) -> (x+y=w367:dbl)
              n259 = script code="Xc=(ximax+ximin)./2;\nYc=(yimax+yimin)./2;\nxout=zeros(size(xin));\nyout=zeros(size(yin));\nfor n=1:length(xin)\nxin(n)=xin(n)-Xc;\nyin(n)=yin(n)-Yc;\nxout(n)=xin(n).*cos(pi/180.*phi)+yin(n).*sin(pi./180.*phi)+Xc;\nyout(n)=-xin(n).*sin(pi./180.*phi)+yin(n).*cos(pi./180.*phi)+Yc;\nend"("??"=w354, "ximax"=w359, "ximin"=w360, "yimax"=w362, "yimin"=w361, "phi"=w367, "xin"=w357, "yin"=w358) -> ("??"=w353:errorcluster, "xout"=w356:dbl[], "yout"=w355:dbl[])
              n260 = local write "X-WaveArray"(w356) -> ()
              n261 = local write "Y-WaveArray"(w355) -> ()
            }
          }
          "error IO" <- w215
          n262 = property on="Scanning Mode" class="Ring (strict)"("Value"=0) -> ()  [unwired: 2 in, 2 out]
        }
        frame 4 {
          n263 = stacked-sequence {
            seq-local: [_ _ _ w423 _] -> [_ _ _ _ w438]
            seq-local: [_ w392 _ _ _] -> [_ _ w417 w424 _]
            seq-local: [w378 _ _ _ _] -> [_ w391 _ _ _]
            seq-local: [w377 _ _ _ _] -> [_ w390 _ _ _]
            seq-local: [w375 _ _ _ _] -> [_ w389 _ _ _]
            seq-local: [w376 _ _ _ _] -> [_ w388 _ _ _]
            tunnel: [_ w392 _ _ _] -> w371
            tunnel: [_ _ _ w422 _] -> w370
            frame #0 {
              # "min"
              # "max"
              n264 = local read "Points"() -> (w379:cluster{"X":dbl, "Y":dbl}[])
              n265 = Array Max & Min(array=w379) -> (max value=w381:cluster{"X":dbl, "Y":dbl}, min value=w380:cluster{"X":dbl, "Y":dbl})  [unwired: 2 out]
              n266 = for {
                tunnel: w379 -> [w387] mode=indexing
                shift-right: [w383] -> w375
                shift-left: 0.0 -> [w386]
                shift-right: [w382] -> w376
                shift-left: 500.0 -> [w384]
                n267 = Unbundle By Name(w387) -> ("Y"=w385:dbl)
                n268 = Max & Min(x=w385, y=w386) -> (max(x,y)=w383:dbl)  [unwired: 1 out]
                n269 = Max & Min(x=w385, y=w384) -> (min(x,y)=w382:dbl)  [unwired: 1 out]
              }
              "max" <- w375
              "min" <- w376
              n270 = Unbundle By Name(w381) -> ("X"=w378:dbl)
              n271 = Unbundle By Name(w380) -> ("X"=w377:dbl)
            }
            frame #1 {
              n272 = local read "Points"() -> (w393:cluster{"X":dbl, "Y":dbl}[])
              n273 = Array Size(array=w393) -> (size(s)=w394:i32)
              n274 = for {
                N: w394 -> [_]
                tunnel: w393 -> [w415] mode=indexing
                tunnel: [w414] -> w392 mode=indexing
                tunnel: w391 -> [w400]
                tunnel: w390 -> [w399]
                tunnel: w389 -> [w398]
                tunnel: w388 -> [w397]
                n275 = Unbundle By Name(w415) -> ("X"=w402:dbl, "Y"=w401:dbl)
                n276 = Subtract(x=w400, y=w399) -> (x-y=w409:dbl)
                n277 = Subtract(x=w402, y=w400) -> (x-y=w410:dbl)
                n278 = Subtract(x=w398, y=w397) -> (x-y=w404:dbl)
                n279 = Subtract(x=w401, y=w398) -> (x-y=w405:dbl)
                n280 = Multiply(x=w410, y=2.0) -> (x*y=w411:dbl)
                n281 = Multiply(x=w405, y=2.0) -> (x*y=w406:dbl)
                n282 = Divide(x=w411, y=w409) -> (x/y=w413:dbl)
                n283 = Divide(x=w406, y=w404) -> (x/y=w407:dbl)
                n284 = Increment(x=w413) -> (x+1=w412:dbl)
                n285 = Increment(x=w407) -> (x+1=w396:dbl)
                n286 = Negate(x=w396) -> (-x=w395:dbl)
                n287 = Bundle(w412, w395) -> (w414:cluster{dbl, dbl})  [unwired: 1 in]
              }
            }
            frame #2 {
              n288 = local read "xPixels/rPixels"() -> (w421:dbl)
              n289 = local read "yPixels/tPixels"() -> (w420:dbl)
              n290 = Array Size(array=w417) -> (size(s)=w418:i32)
              n291 = Multiply(x=w421, y=w420) -> (x*y=w416:dbl)
              n292 = Square(x=w418) -> (x^2=w419:i32)
              n293 = Max & Min(x=w419, y=w416) -> ()  [unwired: 2 out]
              n294 = local write "numPixels"(w416) -> ()
            }
            frame #3 {
              n295 = Array Size(array=w424) -> (size(s)=w425:i32)
              n296 = for {
                N: w425 -> [_]
                tunnel: w424 -> [w435] mode=indexing
                tunnel: [w432] -> w423 mode=indexing
                tunnel: [w431] -> w422 mode=indexing
                n297 = Unbundle(w435) -> (w434:dbl, w433:dbl)
                n298 = Re/Im To Polar(2:w433, 3:w434) -> (0:w426:dbl, 1:w430:dbl)
                n299 = Bundle(w430, w426) -> (w432:cluster{dbl, dbl})  [unwired: 1 in]
                n300 = Compound Arithmetic op=MULTIPLY(w426, 180.0, invert 3.141592653589793) -> (w429:dbl)
                n301 = Bundle(w430, w429) -> (w431:cluster{dbl, dbl})  [unwired: 1 in]
              }
            }
            frame #4 {
              n302 = local read "numPixels"() -> (w439:dbl)
              n303 = for {
                N: w439 -> [w441]
                tunnel: w438 -> [w448]
                tunnel: [w446] -> w437 mode=indexing
                tunnel: [w445] -> w436 mode=indexing
                i -> [w443]
                n304 = Square Root(x=w443) -> (sqrt(x)=w456:dbl)
                n305 = Round Toward -Infinity(1:w456) -> (0:w454:dbl)
                n306 = Square(x=w454) -> (x^2=w455:dbl)
                n307 = Multiply(x=2.0, y=w454) -> (x*y=w453:dbl)
                n308 = Increment(x=w453) -> (x+1=w451:dbl)
                n309 = Subtract(x=w443, y=w455) -> (x-y=w450:dbl)
                n310 = Array Size(array=w448) -> (size(s)=w452:i32)
                n311 = Compound Arithmetic op=MULTIPLY(w452, invert w451, w450) -> (w444:dbl)
                n312 = Round Toward -Infinity(1:w444) -> (0:w442:dbl)
                n313 = Index Array(array=w448, index=w442) -> (element=w457:cluster{dbl, dbl})
                n314 = Decrement(x=w441) -> (x-1=w440:i32)
                n315 = Unbundle(w457) -> (w449:dbl, w446:dbl)
                n316 = Compound Arithmetic op=MULTIPLY(invert w440, w449, w443) -> (w445:dbl)
              }
              n317 = local write "X-WaveArray"(w436) -> ()
              n318 = local write "Y-WaveArray"(w437) -> ()
            }
          }
          n319 = property on="Scanning Mode" class="Ring (strict)"("Value"=u16 1) -> ()  [unwired: 2 in, 2 out]
          n320 = Bundle(w371, w370) -> (w372:T4)  [unwired: 1 in]
          n321 = Unbundle(w372) -> (w369:cluster{dbl, dbl}[])  [unwired: 1 out]
        }
        frame 5 {
          w463 = 6.283185307179586
          n322 = local read "Vx-max"() -> (w475:dbl)
          n323 = local read "Vy-max"() -> (w479:dbl)
          n324 = local read "Vy-max"() -> (w474:dbl)
          n325 = local read "Vx-max"() -> (w486:dbl)
          n326 = local read "Vx-min"() -> (w476:dbl)
          n327 = local read "Vy-min"() -> (w480:dbl)
          n328 = local read "Vy-min"() -> (w473:dbl)
          n329 = local read "Vx-min"() -> (w485:dbl)
          n330 = local read "Angle"() -> (w461:dbl)
          n331 = Subtract(x=w475, y=w476) -> (x-y=w477:dbl)
          n332 = Add(x=w479, y=w480) -> (x+y=w481:dbl)
          n333 = Subtract(x=w474, y=w473) -> (x-y=w472:dbl)
          n334 = Add(x=w486, y=w485) -> (x+y=w484:dbl)
          n335 = Divide(x=w477, y=2.0) -> (x/y=w469:dbl)
          n336 = Divide(x=w481, y=2.0) -> (x/y=w470:dbl)
          n337 = Divide(x=w472, y=2.0) -> (x/y=w468:dbl)
          n338 = Divide(x=w484, y=2.0) -> (x/y=w458:dbl)
          n339 = Compound Arithmetic op=MULTIPLY(w461, invert 360.0, w463) -> (w464:dbl)
          n340 = local read "points in ellipse"() -> (w465:dbl)
          n341 = Quotient & Remainder(x=w464, y=w463) -> (x-y*floor(x/y)=w460:dbl)  [unwired: 1 out]
          n342 = Negate(x=w460) -> (-x=w459:dbl)
          n343 = local write "numPixels"(w465) -> ()
          n344 = script code="t=2*pi*(1:1:N)./N;\nX=A.*cos(t).*cos(phi)-B.*sin(t).*sin(phi)+Xc\nY=A.*cos(t).*sin(phi)+B.*sin(t).*cos(phi)+Yc"("Xc"=w458, "Yc"=w470, "A"=w469, "B"=w468, "phi"=w459, "N"=w465) -> ("X"=w467:dbl[], "Y"=w466:dbl[])  [unwired: 1 in, 1 out]
          n345 = local write "Y-WaveArray"(w466) -> ()
          n346 = local write "X-WaveArray"(w467) -> ()
        }
      }
      "Points 2" <- w1
    }
    frame #1 {
      # "Plotting"
      n347 = local read "Drawing Mode"() -> (w487:u16)
      n348 = case shown="2, 3, 5" w487 {
        frame 0, Default {
          n349 = flat-sequence {
            tunnel: [w493] -> w490
            tunnel: [w494] -> w491
            tunnel: [w519] -> w489
            tunnel: [w520] -> w488
            tunnel: w491 -> [w521]
            tunnel: w490 -> [w522]
            tunnel: w489 -> [w536]
            tunnel: w488 -> [w535]
            frame #0 {
              n350 = local read "Scanning Mode"() -> (w492:u16)
              n351 = case shown="0, Default" w492 {
                tunnel: [w497 w499] -> w493
                tunnel: [w496 w498] -> w494
                frame 0, Default {
                  # "-1<x<1\n-1<y<1"
                  n352 = local read "Y-WaveArray"() -> (w496:dbl[])
                  n353 = local read "X-WaveArray"() -> (w497:dbl[])
                  n354 = Bundle("X-WaveArray"=w497, "Y-WaveArray"=w496) -> (→"X-Y Graph 2":T5)  [unwired: 1 in]
                }
                frame 1 {
                  # "0<x<1\n0<y<2pi"
                  n355 = local read "X-WaveArray"() -> (w500:dbl[])
                  n356 = local read "Y-WaveArray"() -> (w501:dbl[])
                  n357 = Polar To Re/Im(2:w501, 3:w500) -> (0:w498:dbl[], 1:w499:dbl[])
                }
              }
            }
            frame #1 {
              w504 = 2.0
              n358 = local read "Vy-min"() -> (w515:dbl)
              n359 = Subtract(x="Vy-max", y=w515) -> (x-y=w517:dbl)
              n360 = Compound Arithmetic op=MULTIPLY(invert w504, w517, w521) -> (w513:dbl[])
              n361 = local read "Vx-max"() -> (w510:dbl)
              n362 = local read "Vx-min"() -> (w518:dbl)
              n363 = Subtract(x=w510, y=w518) -> (x-y=w516:dbl)
              n364 = Compound Arithmetic op=MULTIPLY(w516, w522, invert w504) -> (w514:dbl[])
              n365 = for {
                tunnel: [w530] -> w512 mode=indexing
                tunnel: [w529] -> w511 mode=indexing
                tunnel: w514 -> [w528] mode=indexing
                tunnel: w513 -> [w527] mode=indexing
                n366 = local read "Angle"() -> (w526:dbl)
                n367 = Compound Arithmetic op=MULTIPLY(6.283185307179586, w526, invert 360.0) -> (w523:dbl)
                n368 = formula code="px = xs*cos(t)+ys*sin(t);\npy = -xs*sin(t)+ys*cos(t);"("xs"=w528, "ys"=w527, "t"=w523) -> ("px"=w530:dbl, "py"=w529:dbl)
              }
              n369 = Add(x="Vy-min", y="Vy-max") -> (x+y=w505:dbl)
              n370 = local read "Vx-min"() -> (w509:dbl)
              n371 = Divide(x=w505, y=w504) -> (x/y=w506:dbl)
              n372 = Add(x=w510, y=w509) -> (x+y=w508:dbl)
              n373 = Add(x=w511, y=w506) -> (x+y=w520:dbl[])
              n374 = Divide(x=w508, y=w504) -> (x/y=w507:dbl)
              n375 = Add(x=w512, y=w507) -> (x+y=w519:dbl[])
            }
            frame #2 {
              n376 = local write "X-WaveArray"(w536) -> ()
              n377 = Bundle(w536, w535) -> (→"X-Y Graph":cluster{dbl[], dbl[]})  [unwired: 1 in]
              n378 = property on="X-Y Graph" class="XYGraph (strict)"("XScale.Maximum"=10.0 ("X Scale.Range:Maximum"), "XScale.Minimum"=-10.0 ("X Scale.Range:Minimum"), "YScale.Maximum"=10.0 ("Y Scale.Range:Maximum"), "YScale.Minimum"=-10.0 ("Y Scale.Range:Minimum")) -> ()  [unwired: 2 in, 2 out]
              n379 = local write "Y-WaveArray"(w535) -> ()
              "X Graph" <- w536
              "Y Graph" <- w535
            }
          }
        }
        frame 2, 3, 5 {
          # "just plotting"
          n380 = local read "Y-WaveArray"() -> (w538:dbl[])
          n381 = local read "X-WaveArray"() -> (w539:dbl[])
          n382 = Bundle("X-WaveArray"=w539, "Y-WaveArray"=w538) -> (w540:T5)  [unwired: 1 in]
          n383 = local write "Y Graph"(w538) -> ()
          n384 = local write "X-Y Graph"(w540) -> ()
          n385 = local write "X Graph"(w539) -> ()
        }
      }
    }
    frame #2 {
      # "smoothing in case any sharp edges"
      n386 = local read "Drawing Mode"() -> (w541:u16)
      n387 = case shown="3" w541 {
        frame 0, Default {
        }
        frame 3 {
          # "interpolates the array"
          # "note- points in ellipse comes from front panel points in contour\n=numPixles"
          # "Draw Freeform"
          n388 = local read "X-WaveArray"() -> (w546:dbl[])
          n389 = local read "points in ellipse"() -> (w561:dbl)
          n390 = local read "Y-WaveArray"() -> (w545:dbl[])
          n391 = Array Size(array=w546) -> (size(s)=w557:i32)
          n392 = local read "points in ellipse"() -> (w553:dbl)
          n393 = Array Size(array=w545) -> (size(s)=w549:i32)
          n394 = Decrement(x=w557) -> (x-1=w556:i32)
          n395 = Decrement(x=w549) -> (x-1=w550:i32)
          n396 = local write "numPixels"(w561) -> ()
          n397 = To Double Precision Float(number=w556) -> (double precision float=w555:dbl)
          n398 = To Double Precision Float(number=w550) -> (double precision float=w551:dbl)
          n399 = Divide(x=w555, y=w561) -> (x/y=w554:dbl)
          n400 = Divide(x=w551, y=w553) -> (x/y=w552:dbl)
          n401 = for {
            N: w561 -> [_]
            tunnel: w546 -> [w612]
            tunnel: w554 -> [w611]
            tunnel: [w610] -> w548 mode=indexing
            i -> [w608]
            n402 = Multiply(x=w611, y=w608) -> (x*y=w609:dbl)
            n403 = Interpolate 1D Array(1:w609, 2:w612) -> (0:w610:dbl)
          }
          n404 = for {
            N: w553 -> [_]
            tunnel: w545 -> [w607]
            tunnel: w552 -> [w606]
            tunnel: [w605] -> w547 mode=indexing
            i -> [w603]
            n405 = Multiply(x=w606, y=w603) -> (x*y=w604:dbl)
            n406 = Interpolate 1D Array(1:w604, 2:w607) -> (0:w605:dbl)
          }
          n407 = Bundle("X-WaveArray"=w546, "Y-WaveArray"=w545) -> (w560:T5)  [unwired: 1 in]
          n408 = disable-structure shown="Disabled" {
            disable-tunnel: [w581 _] -> w559
            disable-tunnel: w548 -> [w577 w602]
            disable-tunnel: w547 -> [w576 w601]
            disable-tunnel: [w563 w602] -> w544
            disable-tunnel: [w562 w601] -> w543
            frame Disabled {
              # "interpolating again...\nbecause previous step might be removing points"
              # "This section tweaks the waveform to reduce acceleration\nbecause 0.00, then a is empty, so this part is disabled"
              # "dr2 = velocity"
              n409 = Rotate 1D Array(1:w577, 2:1 ("n")) -> (0:w589:dbl[])
              n410 = Rotate 1D Array(1:w576, 2:1 ("n")) -> (0:w588:dbl[])
              n411 = Subtract(x=w577, y=w589) -> (x-y=w586:dbl[])
              n412 = Subtract(x=w576, y=w588) -> (x-y=w585:dbl[])
              n413 = Square(x=w586) -> (x^2=w584:dbl[])
              n414 = Square(x=w585) -> (x^2=w583:dbl[])
              n415 = Add(x=w584, y=w583) -> (x+y=w582:dbl[])
              n416 = Square Root(x=w582) -> (sqrt(x)=w580:dbl[])
              "Y Graph 2" <- w580
              n417 = script code="a=dr2<0.00;\nwhile sum(a)>0\nb=diff(a);\nx=x(b<1);\ny=y(b<1);\nx=[x(end) x];\ny=[y(end) y];\ndr2=sqrt((diff(x)).^2+(diff(y)).^ 2)\na=dr2<0.0;\nend\nxout=x;\nyout=y;"("dr2"=w580, "x"=w577, "y"=w576) -> ("xout"=w570:dbl[], "yout"=w564:dbl[])  [unwired: 1 in, 1 out]
              n418 = Bundle(w570, w564) -> (w581:cluster{dbl[], dbl[]})  [unwired: 1 in]
              n419 = Build Array(w577, w570) -> (→"Y Graph 3":dbl[][])
              n420 = Build Array(w576, w564) -> (→"Y Graph 4":dbl[][])
              n421 = local read "points in ellipse"() -> (w565:dbl)
              n422 = local read "points in ellipse"() -> (w575:dbl)
              n423 = Array Size(array=w564) -> (size(s)=w569:i32)
              n424 = Array Size(array=w570) -> (size(s)=w571:i32)
              n425 = Decrement(x=w569) -> (x-1=w568:i32)
              n426 = Decrement(x=w571) -> (x-1=w572:i32)
              n427 = To Double Precision Float(number=w568) -> (double precision float=w567:dbl)
              n428 = To Double Precision Float(number=w572) -> (double precision float=w573:dbl)
              n429 = Divide(x=w567, y=w565) -> (x/y=w566:dbl)
              n430 = Divide(x=w573, y=w575) -> (x/y=w574:dbl)
              n431 = for {
                N: w565 -> [_]
                tunnel: w564 -> [w595]
                tunnel: w566 -> [w594]
                tunnel: [w593] -> w562 mode=indexing
                i -> [w591]
                n432 = Multiply(x=w594, y=w591) -> (x*y=w592:dbl)
                n433 = Interpolate 1D Array(1:w592, 2:w595) -> (0:w593:dbl)
              }
              n434 = for {
                N: w575 -> [_]
                tunnel: w570 -> [w600]
                tunnel: w574 -> [w599]
                tunnel: [w598] -> w563 mode=indexing
                i -> [w596]
                n435 = Multiply(x=w599, y=w596) -> (x*y=w597:dbl)
                n436 = Interpolate 1D Array(1:w597, 2:w600) -> (0:w598:dbl)
              }
            }
            frame Enabled {
            }
          }
          n437 = local write "Y-WaveArray"(w543) -> ()
          n438 = local write "X-WaveArray"(w544) -> ()
          n439 = Bundle(w544, w543) -> (w542:cluster{dbl[], dbl[]})  [unwired: 1 in]
          n440 = Build Array(w560, w559, w542) -> (→"X-Y Graph 3":T1)
        }
      }
    }
  }
